vi "Write Sample Metadata.vi"(0 "File Path":path, 11 "Error In":errorcluster) -> (4 "File Path (Dup)":path, 8 "Canceled?":bool, 15 "Write Error":errorcluster)   [LabVIEW 2016]
uses:
  <vilib>/Utility/miscctls.llb/LVPointTypeDef.ctl
  Sampel Metadata Type Defs/Sample Metadata Full Data.ctl
  Sampel Metadata Type Defs/Sample Metadata Name Value Pair.ctl
  Sampel Metadata Type Defs/Sample Metadata Probe Data.ctl
  <vilib>/regexp/Match Regular Expression.xnode
  shell32.dll
panel:
  out "Current Path":string
  out "Last File Write Error":errorcluster
  in  "Dirty Quit":bool
  in  "Scavenger 06":u16(ring) items=["Not Applicable", "-", "Add Item"]
  in  "Scavenger 05":u16(ring) items=["Not Applicable", "-", "Add Item"]
  in  "Scavenger 04":u16(ring) items=["Not Applicable", "-", "Add Item"]
  in  "Scavenger 03":u16(ring) items=["Not Applicable", "-", "Add Item"]
  in  "Scavenger 02":u16(ring) items=["Not Applicable", "-", "Add Item"]
  in  "Scavenger 01":u16(ring) items=["Not Applicable", "-", "Add Item"]
  in  "Load Preset":bool
  in  "Sealant":u16(ring) items=["Not Applicable", "-", "Add Item"]
  in  "Sample Holder":u16(ring) items=["Not Applicable", "-", "Add Item"]
  in  "Preset Metadata":u16(ring) items=["None"]
  in  "Save New Preset":bool
  in  "Notes":string caption="Additional Notes (e.g. fixation info)"
  in  "Extra Tag 06":u16(ring) caption="Extra Tag" items=["Not Applicable", "-", "Add Item"]
  in  "Extra Tag 05":u16(ring) caption="Extra Tag" items=["Not Applicable", "-", "Add Item"]
  in  "Extra Tag 04":u16(ring) caption="Extra Tag" items=["Not Applicable", "-", "Add Item"]
  in  "Extra Tag 03":u16(ring) caption="Extra Tag" items=["Not Applicable", "-", "Add Item"]
  in  "Extra Tag 02":u16(ring) caption="Extra Tag" items=["Not Applicable", "-", "Add Item"]
  in  "Extra Tag 01":u16(ring) caption="Extra Tag" items=["Not Applicable", "-", "Add Item"]
  in  "Image Target 04":u16(ring) caption="Image Target" items=["Not Applicable", "-", "Add Item"]
  in  "Image Target 03":u16(ring) caption="Image Target" items=["Not Applicable", "-", "Add Item"]
  in  "Image Target 02":u16(ring) caption="Image Target" items=["Not Applicable", "-", "Add Item"]
  in  "Image Target 01":u16(ring) caption="Probe Target" items=["Not Applicable", "-", "Add Item"]
  in  "Buffer PH":dbl=1.0 caption="PH"
  in  "Buffer Type":u16(ring) items=["Not Applicable", "-", "Add Item"]
  in  "Probe Concentration 04":dbl=1.0 caption="Concentration"
  in  "Probe Concentration 03":dbl=1.0 caption="Concentration"
  in  "Probe Concentration 02":dbl=1.0 caption="Concentration"
  in  "Probe Concentration 01":dbl=1.0 caption="Concentration"
  in  "Probe Cat Num 04":u16(ring) caption="Probe Cat Num" items=["Not Applicable", "-", "Add Item"]
  in  "Probe Sub Type 04":u16(ring) caption="Probe Sub Type" items=["Not Applicable", "-", "Add Item"]
  in  "Probe Name 04":u16(ring) caption="Probe Name" items=["Not Applicable", "-", "Add Item"]
  in  "Probe 4":bool
  in  "Probe Cat Num 03":u16(ring) caption="Probe Cat Num" items=["Not Applicable", "-", "Add Item"]
  in  "Probe Cat Num 02":u16(ring) caption="Probe Cat Num" items=["Not Applicable", "-", "Add Item"]
  in  "Probe Cat Num 01":u16(ring) caption="Catalog Number" items=["Not Applicable", "-", "Add Item"]
  in  "Probe Sub Type 03":u16(ring) caption="Probe Sub Type" items=["Not Applicable", "-", "Add Item"]
  in  "Probe Sub Type 02":u16(ring) caption="Probe Sub Type" items=["Not Applicable", "-", "Add Item"]
  in  "Probe Sub Type 01":u16(ring) caption="Probe Sub Type" items=["Not Applicable", "-", "Add Item"]
  in  "Probe Name 03":u16(ring) caption="Probe Name" items=["Not Applicable", "-", "Add Item"]
  in  "Probe Name 02":u16(ring) caption="Probe Name" items=["Not Applicable", "-", "Add Item"]
  in  "Probe Name 01":u16(ring) caption="Probe Name" items=["Not Applicable", "-", "Add Item"]
  in  "Probe 3":bool
  in  "Probe 2":bool
  in  "Probe 1":bool
  in  "Sample Type Sub Types":u16(ring) caption="Sample Sub Type" items=["Not Applicable", "-", "Add Item"]
  in  "Sample Type":u16(ring) items=["Not Applicable", "-", "Add Item"]
  in  "Cancel":bool
  in  "Save":bool
  # "Sample Type"
  # "Sample Mounting"
  # "Buffer Information"
  # "Oxygen Scavenger Components"
  # "Probe Information"
  # "Probe Active"
  # "Additional Tags"
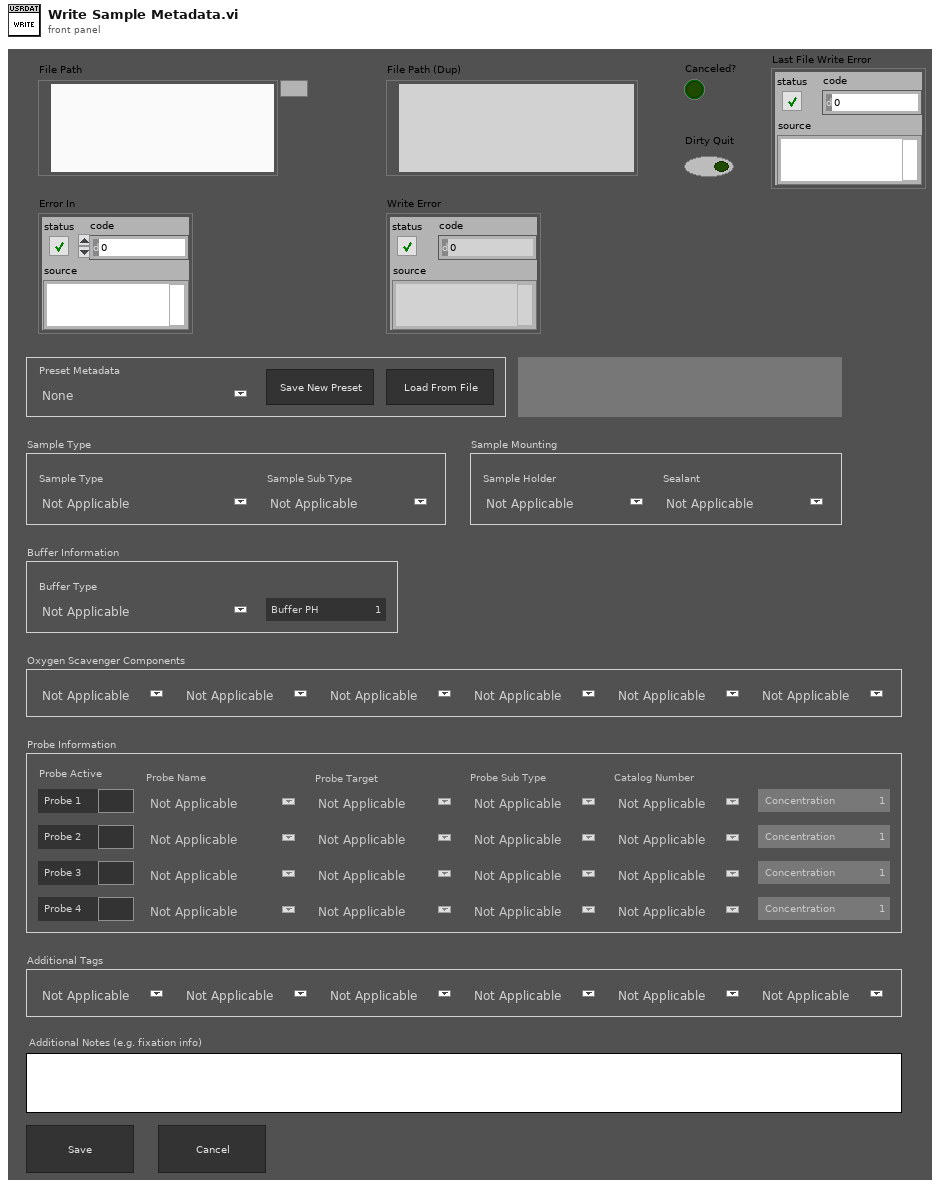
[diagram p1: front panel]
types:
  T1 = typedef "Sample Metadata Full Data.ctl" = cluster{"Sample Type":T2, "Sample Sub Type":T2, "Proble Data":T3[], "Buffer Type":T2, "Oxygen Scavenger":T2, "Buffer PH":dbl, "Extra Tags":T2[], "Sample Holder":T2, "Sealant":T2, "Notes":string, "Preset Name":string, "Scavenger Tags":T2[]}
  T2 = typedef "Sample Metadata Name Value Pair.ctl" = cluster{"String":string, "Value":u16}
  T3 = typedef "Sample Metadata Probe Data.ctl" = cluster{"Active?":bool, "Name":T2, "Target":T2, "Sub Type":T2, "Cat Number":T2, "Concentration":dbl}
  T4 = enum16{"Always On", "Always Off", "Off While Running"}
  T5 = typedef "LVPointTypeDef.ctl" = cluster{"Horizontal":i16, "Vertical":i16}
  T6 = enum8{"Enabled", "Disabled", "Disabled and Grayed Out"}
  T7 = typedef "LVRectTypeDef.ctl" = cluster{"Left":i16, "Top":i16, "Right":i16, "Bottom":i16}
  T8 = typedef "LVBoundsTypeDef.ctl" = cluster{"Width":u32, "Height":u32}
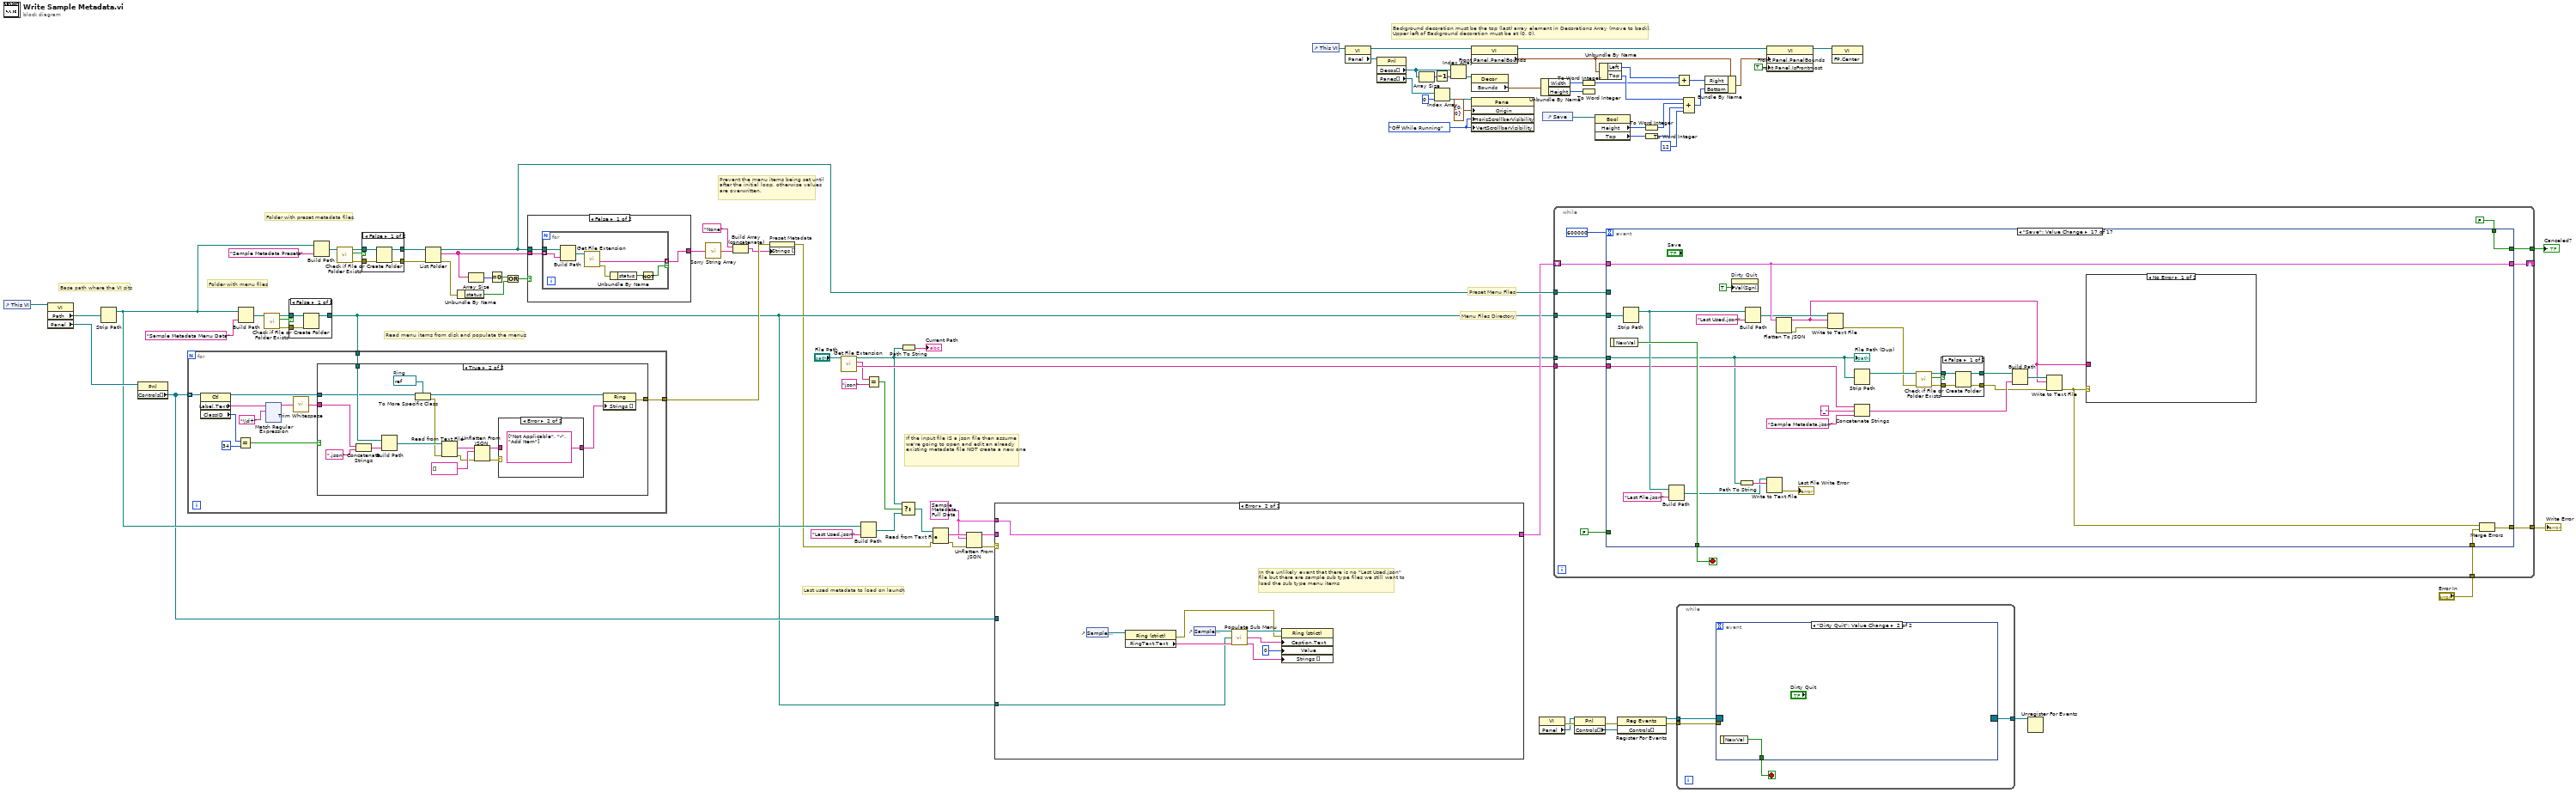
[diagram p0: block diagram]
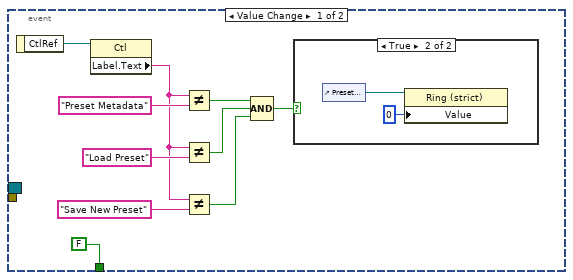
[diagram p2: hidden frame]
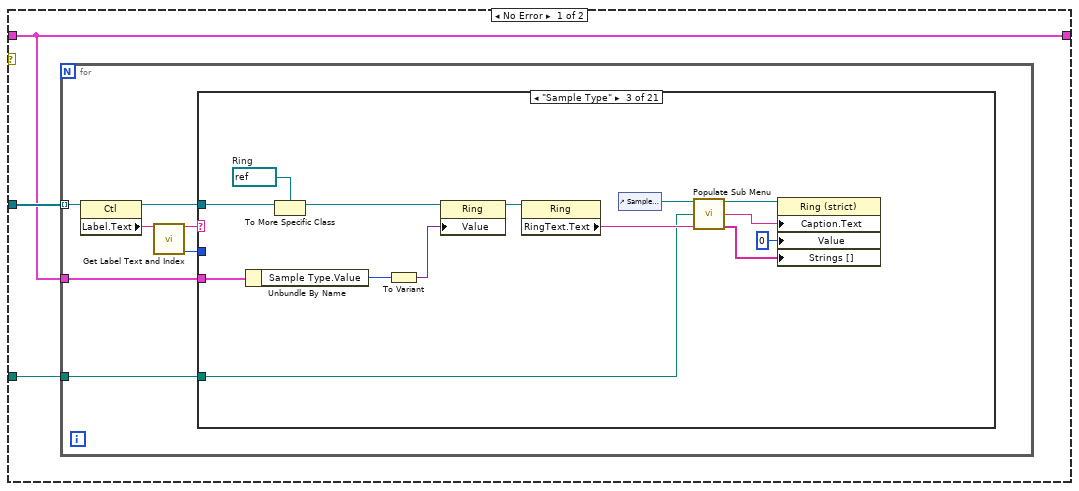
[diagram p4: hidden frame]
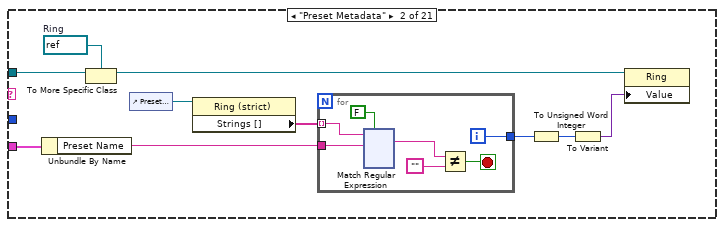
[diagram p6: hidden frame]
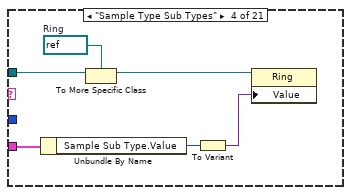
[diagram p7: hidden frame]
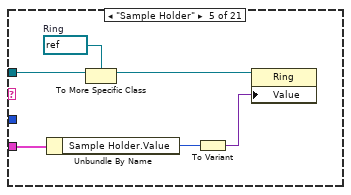
[diagram p8: hidden frame]
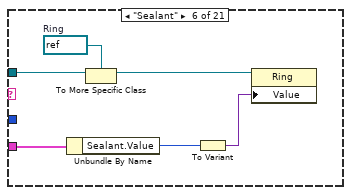
[diagram p9: hidden frame]
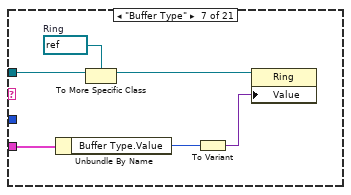
[diagram p10: hidden frame]
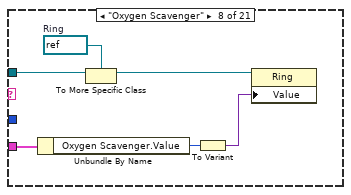
[diagram p11: hidden frame]
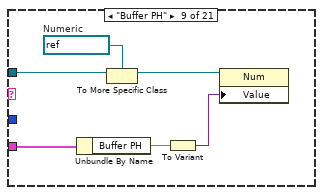
[diagram p12: hidden frame]
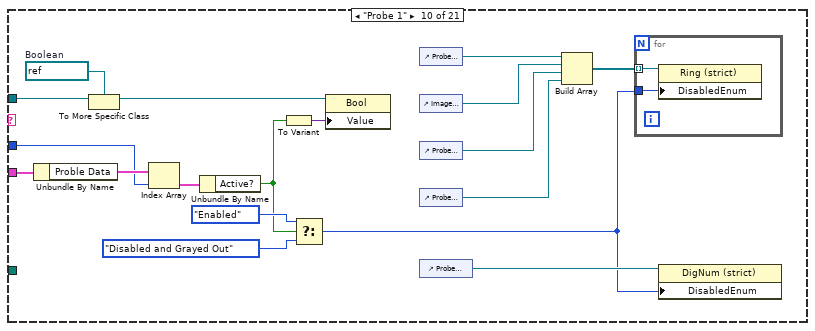
[diagram p13: hidden frame]
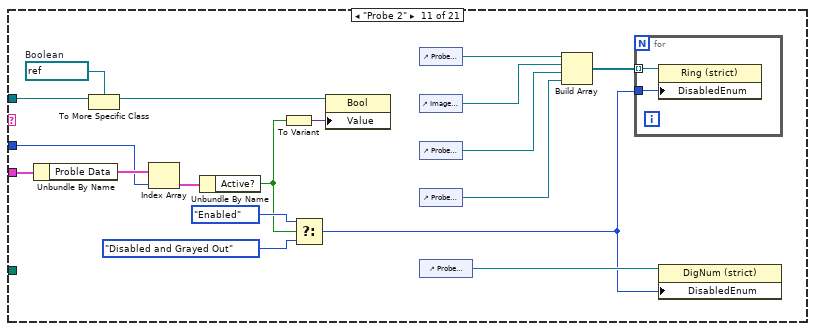
[diagram p14: hidden frame]
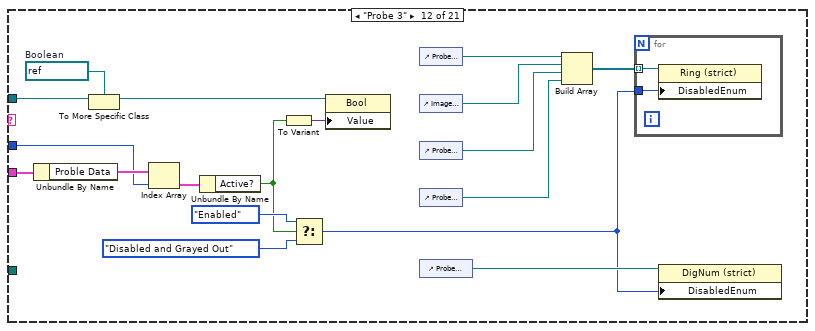
[diagram p15: hidden frame]
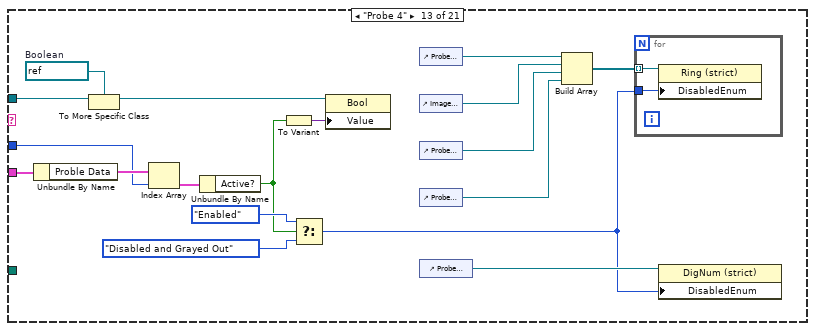
[diagram p16: hidden frame]
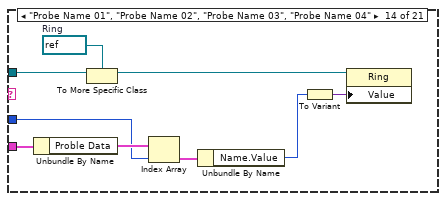
[diagram p17: hidden frame]
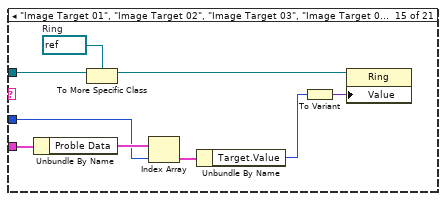
[diagram p18: hidden frame]
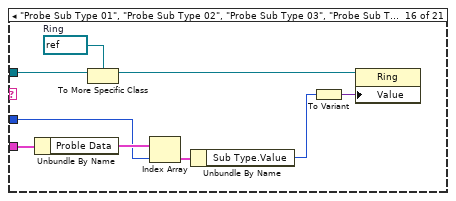
[diagram p19: hidden frame]
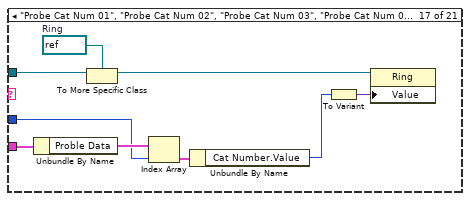
[diagram p20: hidden frame]
diagram:
  w29 = T1 {"Sample Type"={"String"="", "Value"=0}, "Sample Sub Type"={"String"="", "Value"=0}, "Proble Data"=[{"Active?"=FALSE, "Name"={"String"="", "Value"=0}, "Target"={"String"="", "Value"=0}, "Sub Type"={"String"="", "Value"=0}, "Cat Number"={"String"="", "Value"=0}, "Concentration"=0.0}, {"Active?"=FALSE, "Name"={"String"="", "Value"=0}, "Target"={"String"="", "Value"=0}, "Sub Type"={"String"="", "Value"=0}, "Cat Number"={"String"="", "Value"=0}, "Concentration"=0.0}, {"Active?"=FALSE, "Name"={"String"="", "Value"=0}, "Target"={"String"="", "Value"=0}, "Sub Type"={"String"="", "Value"=0}, "Cat Number"={"String"="", "Value"=0}, "Concentration"=0.0}, {"Active?"=FALSE, "Name"={"String"="", "Value"=0}, "Target"={"String"="", "Value"=0}, "Sub Type"={"String"="", "Value"=0}, "Cat Number"={"String"="", "Value"=0}, "Concentration"=0.0}], "Buffer Type"={"String"="", "Value"=0}, "Oxygen Scavenger"={"String"="", "Value"=0}, "Buffer PH"=0.0, "Extra Tags"=[{"String"="", "Value"=0}, {"String"="", "Value"=0}, {"String"="", "Value"=0}, {"String"="", "Value"=0}, {"String"="", "Value"=0}, {"String"="", "Value"=0}], "Sample Holder"={"String"="", "Value"=0}, "Sealant"={"String"="", "Value"=0}, "Notes"="", "Preset Name"="", "Scavenger Tags"=[{"String"="", "Value"=0}, {"String"="", "Value"=0}, {"String"="", "Value"=0}, {"String"="", "Value"=0}, {"String"="", "Value"=0}, {"String"="", "Value"=0}]} ("Sample Metadata")
  w71 = T4."Off While Running" ("Vertical Scrollbar Visibility")
  # "If the input file IS a json file then assume we're going to open and edit an already existing metadata file NOT create a new one"
  # "Last used metadata to load on launch"
  # "Preset Menu Files"
  # "Menu Files Directory"
  # "Prevent the menu items being set until after the initial loop, otherwise values are overwritten."
  # "Folder with preset metadata files"
  # "Folder with menu files"
  # "Read menu items from disk and populate the menus"
  # "Base path where the VI sits"
  # "Background decoration must be the top (last) array element in Decorations Array (move to back).\nUpper left of Background decoration must be at (0, 0)."
  n1 = control-ref of="This VI"() -> (w57:refnum<vi>)
  n2 = property class="VI"(reference=w57) -> ("Path"=w34:path, "Panel"=w55:refnum<vi>)  [unwired: 1 in, 2 out]
  n3 = Strip Path(path=w34) -> (stripped path=w33:path)  [unwired: 1 out]
  n4 = property class="Pnl"(reference=w55) -> ("Controls[]"=w28:refnum<vi>[])  [unwired: 1 in, 2 out]
  n5 = Build Path(base path=w33, name or relative path="Sample Metadata Menu Data") -> (appended path=w53:path)
  n6 = call <vilib>:"Check if File or Folder Exists.vi"("path"=w53) -> ("error out"=w38:errorcluster, "file or folder exists?"=w51:bool, "dup path"=w52:path)  [unwired: 8 in]
  n7 = case shown="False" w51 {
    tunnel: w52 -> [w91 w92]
    tunnel: [w90 w92] -> w26
    tunnel: w38 -> [w89 _]
    frame False {
      n8 = Create Folder(path (use dialog)=w91, error in=w89) -> (created path=w90:path)  [unwired: 1 in, 2 out]
    }
    frame True {
    }
  }
  n9 = for {
    tunnel: w28 -> [w103] mode=indexing
    tunnel: w26 -> [w99]
    tunnel: [w93] -> w37
    n10 = property class="Ctl"(reference=w103) -> (reference out=w101:refnum<vi>, "Label.Text"=w96:string, "ClassID"=w100:u32)  [unwired: 1 in, 1 out]
    n11 = Equal?(x=w100, y=u32 34) -> (x = y?=w102:bool)
    n12 = xnode "Match Regular Expression"("input string"=w96, "regular expression"="\\d+") -> ("before match"=w98:string)  [unwired: 4 in, 4 out]
    n13 = call <vilib>:"Trim Whitespace.vi"("string"=w98) -> ("trimmed string"=w95:string)  [unwired: 1 in]
    n14 = case shown="True" w102 {
      tunnel: w101 -> [_ w224]
      tunnel: w95 -> [_ w232]
      tunnel: w99 -> [_ w231]
      tunnel: [errorcluster {"status"=FALSE, "code"=0, "source"=""} ("error out") w219] -> w93
      frame False {
      }
      frame True {
        w223 = refnum<vi> refnum  # Ring
        n15 = Concatenate Strings(w232, ".json") -> (w233:string)
        n16 = Build Path(base path=w231, name or relative path=w233) -> (appended path=w230:path)
        n17 = To More Specific Class(target class=w223, reference=w224) -> (specific class reference=w222:refnum<vi>, error out=w220:errorcluster)  [unwired: 1 in]
        n18 = Read from Text File(file (use dialog)=w230, error in=w220) -> (text=w229:string, error out=w227:errorcluster)  [unwired: 2 in, 2 out]
        n19 = Unflatten From JSON(JSON string=w229, type and defaults=string[] [], error in (no error)=w227) -> (value=w225:string[], error out=w226:errorcluster)  [unwired: 4 in]
        n20 = case shown="Error" w226 {
          tunnel: w225 -> [w235 _]
          tunnel: [w235 string[] ["Not Applicable", "-", "Add Item"]] -> w221
          frame No Error {
          }
          frame Error {
          }
        }
        n21 = property class="Ring"(reference=w222, "Strings []"=w221) -> (error out=w219:errorcluster)  [unwired: 1 in, 1 out]
      }
    }
  }
  n22 = Build Path(base path=w33, name or relative path="Sample Metadata Presets") -> (appended path=w48:path)
  n23 = call <vilib>:"Check if File or Folder Exists.vi"("path"=w48) -> ("error out"=w40:errorcluster, "file or folder exists?"=w50:bool, "dup path"=w49:path)  [unwired: 8 in]
  n24 = case shown="False" w50 {
    tunnel: w49 -> [w240 w242]
    tunnel: [w239 w242] -> w47
    tunnel: w40 -> [w238 w241]
    tunnel: [w237 w241] -> w39
    frame False {
      n25 = Create Folder(path (use dialog)=w240, error in=w238) -> (created path=w239:path, error out=w237:errorcluster)  [unwired: 1 in, 1 out]
    }
    frame True {
    }
  }
  n26 = List Folder(path=w47, error in=w39) -> (path out=w36:path, filenames=w45:string[], error out=w46:errorcluster)  [unwired: 2 in, 1 out]
  n27 = Unbundle By Name(w46) -> ("status"=w42:bool)
  n28 = Array Size(array=w45) -> (size(s)=w44:i32)
  n29 = Equal To 0?(x=w44) -> (x = 0?=w43:bool)
  n30 = Or(x=w43, y=w42) -> (x .or. y?=w41:bool)
  n31 = case shown="False" w41 {
    tunnel: w45 -> [w245 _]
    tunnel: [w243 string[] []] -> w22
    tunnel: w36 -> [w244 _]
    frame False {
      n32 = for {
        tunnel: w245 -> [w251] mode=indexing
        tunnel: w244 -> [w252]
        tunnel: [w249] -> w243 mode=indexing if=w246
        n33 = Build Path(base path=w252, name or relative path=w251) -> (appended path=w250:path)
        n34 = call <vilib>:"Get File Extension.vi"("file"=w250) -> ("error out"=w248:errorcluster, "filename without extension"=w249:string)  [unwired: 6 in, 3 out]
        n35 = Unbundle By Name(w248) -> ("status"=w247:bool)
        n36 = Not(x=w247) -> (.not. x?=w246:bool)
      }
    }
    frame True {
    }
  }
  n37 = call "Sorry String Array.vi"("Array of String"=w22) -> ("Sorted Array"=w21:string[])  [unwired: 14 in]
  n38 = Build Array (concatenate)("None", w21) -> (w19:string[])
  n39 = property on="Preset Metadata" class="Ring (strict)"(error in=w37, "Strings []"=w19) -> (error out=w18:errorcluster)  [unwired: 1 in, 1 out]
  n40 = call <vilib>:"Get File Extension.vi"("file"="File Path") -> ("filename without extension"=w8:string, "lowercase file extension"=w7:string, "dup file"=w2:path)  [unwired: 6 in, 2 out]
  n41 = Build Path(base path=w33, name or relative path="Last Used.json") -> (appended path=w4:path)
  n42 = Equal?(x=w7, y="json") -> (x = y?=w5:bool)
  n43 = Select(t=w2, s=w5, f=w4) -> (s? t:f=w3:path)
  n44 = Path To String(path=w2) -> (string=→"Current Path":string)
  n45 = Read from Text File(file (use dialog)=w3, error in=w18) -> (text=w32:string, error out=w17:errorcluster)  [unwired: 2 in, 2 out]
  n46 = Unflatten From JSON(JSON string=w32, type and defaults=w29, error in (no error)=w17) -> (value=w30:T1, error out=w31:errorcluster)  [unwired: 4 in]
  n47 = case shown="Error" w31 {
    tunnel: [w254 w602] -> w27
    tunnel: w28 -> [w256 _]
    tunnel: w26 -> [w255 w594]
    tunnel: w30 -> [w254 _]
    tunnel: w29 -> [_ w602]
    frame No Error {
      n48 = for {
        tunnel: w256 -> [w263] mode=indexing
        tunnel: w254 -> [w261]
        tunnel: w255 -> [w260]
        n49 = property class="Ctl"(reference=w263) -> (reference out=w262:refnum<vi>, "Label.Text"=w259:string)  [unwired: 1 in, 1 out]
        n50 = call "Get Label Text and Index.vi"("Label Text and Index"=w259) -> ("Label Text and Index (Dup)"=w258:string, "Index"=w257:i32)  [unwired: 12 in, 1 out]
        n51 = case shown="\"Sample Type\"" w258 {
          tunnel: w262 -> [_ w272 w407 w413 w419 w425 w431 w437 w443 w458 w478 w498 w518 w530 w539 w548 w557 w566 w575 w584 w590]
          tunnel: w261 -> [_ w270 w405 w411 w417 w423 w429 w435 w441 w462 w482 w502 w522 w533 w542 w551 w560 w569 w578 w587 w589]
          tunnel: w260 -> [_ _ w395 _ _ _ _ _ _ _ _ _ _ _ _ _ _ _ _ _ _]
          tunnel: w257 -> [_ _ _ _ _ _ _ _ _ w445 w465 w485 w505 w525 w534 w543 w552 w561 w570 w579 _]
          frame Default {
          }
          frame "Preset Metadata" {
            w273 = refnum<vi> refnum  # Ring
            n52 = Unbundle By Name(w270) -> ("Preset Name"=w265:string)
            n53 = To More Specific Class(target class=w273, reference=w272) -> (specific class reference=w271:refnum<vi>)  [unwired: 1 in, 1 out]
            n54 = control-ref of="Preset Metadata"() -> (w267:refnum<vi>)
            n55 = property class="Ring (strict)"(reference=w267) -> ("Strings []"=w268:string[])  [unwired: 1 in, 2 out]
            n56 = for {
              tunnel: w265 -> [w280]
              tunnel: w268 -> [w278] mode=indexing
              tunnel: [w274] -> w266
              i -> [w274]
              stop <- w277 stop-if-true
              n57 = xnode "Match Regular Expression"("input string"=w278, "regular expression"=w280, "ignore case? (F)"=FALSE) -> ("whole match"=w276:string)  [unwired: 3 in, 4 out]
              n58 = Not Equal?(x=w276, y="") -> (x != y?=w277:bool)
            }
            n59 = To Unsigned Word Integer(number=w266) -> (unsigned 16bit integer=w264:u16)
            n60 = To Variant(anything=w264) -> (Variant=w269:variant)
            n61 = property class="Ring"(reference=w271, "Value"=w269) -> ()  [unwired: 1 in, 2 out]
          }
          frame "Sample Type" {
            w408 = refnum<vi> refnum  # Ring
            n62 = Unbundle By Name(w405) -> ("Sample Type.Value"=w404:u16)
            n63 = To More Specific Class(target class=w408, reference=w407) -> (specific class reference=w406:refnum<vi>)  [unwired: 1 in, 1 out]
            n64 = To Variant(anything=w404) -> (Variant=w403:variant)
            n65 = property class="Ring"(reference=w406, "Value"=w403) -> (reference out=w402:refnum<vi>)  [unwired: 1 in, 1 out]
            n66 = property class="Ring"(reference=w402) -> ("RingText.Text"=w396:string)  [unwired: 1 in, 2 out]
            n67 = control-ref of="Sample Type Sub Types"() -> (w400:refnum<vi>)
            n68 = call "Populate Sub Menu.vi"("Sample Type Sub Types"=w400, "Base Path"=w395, "Ring Text"=w396) -> ("Sample Type Sub Types (Dup)"=w399:refnum<vi>, "Caption Text"=w398:string, "Menu Items"=w397:string[])  [unwired: 10 in]
            n69 = property class="Ring (strict)"(reference=w399, "Caption.Text"=w398, "Value"=u16 0, "Strings []"=w397) -> ()  [unwired: 1 in, 2 out]
          }
          frame "Sample Type Sub Types" {
            w414 = refnum<vi> refnum  # Ring
            n70 = Unbundle By Name(w411) -> ("Sample Sub Type.Value"=w410:u16)
            n71 = To More Specific Class(target class=w414, reference=w413) -> (specific class reference=w412:refnum<vi>)  [unwired: 1 in, 1 out]
            n72 = To Variant(anything=w410) -> (Variant=w409:variant)
            n73 = property class="Ring"(reference=w412, "Value"=w409) -> ()  [unwired: 1 in, 2 out]
          }
          frame "Sample Holder" {
            w420 = refnum<vi> refnum  # Ring
            n74 = Unbundle By Name(w417) -> ("Sample Holder.Value"=w416:u16)
            n75 = To More Specific Class(target class=w420, reference=w419) -> (specific class reference=w418:refnum<vi>)  [unwired: 1 in, 1 out]
            n76 = To Variant(anything=w416) -> (Variant=w415:variant)
            n77 = property class="Ring"(reference=w418, "Value"=w415) -> ()  [unwired: 1 in, 2 out]
          }
          frame "Sealant" {
            w426 = refnum<vi> refnum  # Ring
            n78 = Unbundle By Name(w423) -> ("Sealant.Value"=w422:u16)
            n79 = To More Specific Class(target class=w426, reference=w425) -> (specific class reference=w424:refnum<vi>)  [unwired: 1 in, 1 out]
            n80 = To Variant(anything=w422) -> (Variant=w421:variant)
            n81 = property class="Ring"(reference=w424, "Value"=w421) -> ()  [unwired: 1 in, 2 out]
          }
          frame "Buffer Type" {
            w432 = refnum<vi> refnum  # Ring
            n82 = Unbundle By Name(w429) -> ("Buffer Type.Value"=w428:u16)
            n83 = To More Specific Class(target class=w432, reference=w431) -> (specific class reference=w430:refnum<vi>)  [unwired: 1 in, 1 out]
            n84 = To Variant(anything=w428) -> (Variant=w427:variant)
            n85 = property class="Ring"(reference=w430, "Value"=w427) -> ()  [unwired: 1 in, 2 out]
          }
          frame "Oxygen Scavenger" {
            w438 = refnum<vi> refnum  # Ring
            n86 = Unbundle By Name(w435) -> ("Oxygen Scavenger.Value"=w434:u16)
            n87 = To More Specific Class(target class=w438, reference=w437) -> (specific class reference=w436:refnum<vi>)  [unwired: 1 in, 1 out]
            n88 = To Variant(anything=w434) -> (Variant=w433:variant)
            n89 = property class="Ring"(reference=w436, "Value"=w433) -> ()  [unwired: 1 in, 2 out]
          }
          frame "Buffer PH" {
            w444 = refnum<vi> refnum  # Numeric
            n90 = Unbundle By Name(w441) -> ("Buffer PH"=w440:dbl)
            n91 = To More Specific Class(target class=w444, reference=w443) -> (specific class reference=w442:refnum<vi>)  [unwired: 1 in, 1 out]
            n92 = To Variant(anything=w440) -> (Variant=w439:variant)
            n93 = property class="Num"(reference=w442, "Value"=w439) -> ()  [unwired: 1 in, 2 out]
          }
          frame "Probe 1" {
            w459 = refnum<vi> refnum  # Boolean
            n94 = Unbundle By Name(w462) -> ("Proble Data"=w461:T3[])
            n95 = To More Specific Class(target class=w459, reference=w458) -> (specific class reference=w457:refnum<vi>)  [unwired: 1 in, 1 out]
            n96 = Index Array(array=w461, index=w445) -> (element=w460:T3)
            n97 = Unbundle By Name(w460) -> ("Active?"=w447:bool)
            n98 = To Variant(anything=w447) -> (Variant=w456:variant)
            n99 = Select(t=T6."Enabled" ("Disabled"), s=w447, f=T6."Disabled and Grayed Out" ("Disabled")) -> (s? t:f=w446:T6)
            n100 = property class="Bool"(reference=w457, "Value"=w456) -> ()  [unwired: 1 in, 2 out]
            n101 = control-ref of="Probe Name 01"() -> (w452:refnum<vi>)
            n102 = control-ref of="Image Target 01"() -> (w453:refnum<vi>)
            n103 = control-ref of="Probe Sub Type 01"() -> (w454:refnum<vi>)
            n104 = control-ref of="Probe Cat Num 01"() -> (w455:refnum<vi>)
            n105 = control-ref of="Probe Concentration 01"() -> (w450:refnum<vi>)
            n106 = Build Array(w452, w453, w454, w455) -> (w451:refnum<vi>[])
            n107 = for {
              tunnel: w451 -> [w464] mode=indexing
              tunnel: w446 -> [w463]
              n108 = property class="Ring (strict)"(reference=w464, "DisabledEnum"=w463) -> ()  [unwired: 1 in, 2 out]
            }
            n109 = property class="DigNum (strict)"(reference=w450, "DisabledEnum"=w446) -> ()  [unwired: 1 in, 2 out]
          }
          frame "Probe 2" {
            w479 = refnum<vi> refnum  # Boolean
            n110 = Unbundle By Name(w482) -> ("Proble Data"=w481:T3[])
            n111 = To More Specific Class(target class=w479, reference=w478) -> (specific class reference=w477:refnum<vi>)  [unwired: 1 in, 1 out]
            n112 = Index Array(array=w481, index=w465) -> (element=w480:T3)
            n113 = Unbundle By Name(w480) -> ("Active?"=w467:bool)
            n114 = To Variant(anything=w467) -> (Variant=w476:variant)
            n115 = Select(t=T6."Enabled" ("Disabled"), s=w467, f=T6."Disabled and Grayed Out" ("Disabled")) -> (s? t:f=w466:T6)
            n116 = property class="Bool"(reference=w477, "Value"=w476) -> ()  [unwired: 1 in, 2 out]
            n117 = control-ref of="Probe Name 02"() -> (w472:refnum<vi>)
            n118 = control-ref of="Image Target 02"() -> (w473:refnum<vi>)
            n119 = control-ref of="Probe Sub Type 02"() -> (w474:refnum<vi>)
            n120 = control-ref of="Probe Cat Num 02"() -> (w475:refnum<vi>)
            n121 = control-ref of="Probe Concentration 02"() -> (w470:refnum<vi>)
            n122 = Build Array(w472, w473, w474, w475) -> (w471:refnum<vi>[])
            n123 = for {
              tunnel: w471 -> [w484] mode=indexing
              tunnel: w466 -> [w483]
              n124 = property class="Ring (strict)"(reference=w484, "DisabledEnum"=w483) -> ()  [unwired: 1 in, 2 out]
            }
            n125 = property class="DigNum (strict)"(reference=w470, "DisabledEnum"=w466) -> ()  [unwired: 1 in, 2 out]
          }
          frame "Probe 3" {
            w499 = refnum<vi> refnum  # Boolean
            n126 = Unbundle By Name(w502) -> ("Proble Data"=w501:T3[])
            n127 = To More Specific Class(target class=w499, reference=w498) -> (specific class reference=w497:refnum<vi>)  [unwired: 1 in, 1 out]
            n128 = Index Array(array=w501, index=w485) -> (element=w500:T3)
            n129 = Unbundle By Name(w500) -> ("Active?"=w487:bool)
            n130 = To Variant(anything=w487) -> (Variant=w496:variant)
            n131 = Select(t=T6."Enabled" ("Disabled"), s=w487, f=T6."Disabled and Grayed Out" ("Disabled")) -> (s? t:f=w486:T6)
            n132 = property class="Bool"(reference=w497, "Value"=w496) -> ()  [unwired: 1 in, 2 out]
            n133 = control-ref of="Probe Name 03"() -> (w492:refnum<vi>)
            n134 = control-ref of="Image Target 03"() -> (w493:refnum<vi>)
            n135 = control-ref of="Probe Sub Type 03"() -> (w494:refnum<vi>)
            n136 = control-ref of="Probe Cat Num 03"() -> (w495:refnum<vi>)
            n137 = control-ref of="Probe Concentration 03"() -> (w490:refnum<vi>)
            n138 = Build Array(w492, w493, w494, w495) -> (w491:refnum<vi>[])
            n139 = for {
              tunnel: w491 -> [w504] mode=indexing
              tunnel: w486 -> [w503]
              n140 = property class="Ring (strict)"(reference=w504, "DisabledEnum"=w503) -> ()  [unwired: 1 in, 2 out]
            }
            n141 = property class="DigNum (strict)"(reference=w490, "DisabledEnum"=w486) -> ()  [unwired: 1 in, 2 out]
          }
          frame "Probe 4" {
            w519 = refnum<vi> refnum  # Boolean
            n142 = Unbundle By Name(w522) -> ("Proble Data"=w521:T3[])
            n143 = To More Specific Class(target class=w519, reference=w518) -> (specific class reference=w517:refnum<vi>)  [unwired: 1 in, 1 out]
            n144 = Index Array(array=w521, index=w505) -> (element=w520:T3)
            n145 = Unbundle By Name(w520) -> ("Active?"=w507:bool)
            n146 = To Variant(anything=w507) -> (Variant=w516:variant)
            n147 = Select(t=T6."Enabled" ("Disabled"), s=w507, f=T6."Disabled and Grayed Out" ("Disabled")) -> (s? t:f=w506:T6)
            n148 = property class="Bool"(reference=w517, "Value"=w516) -> ()  [unwired: 1 in, 2 out]
            n149 = control-ref of="Probe Name 04"() -> (w512:refnum<vi>)
            n150 = control-ref of="Image Target 04"() -> (w513:refnum<vi>)
            n151 = control-ref of="Probe Sub Type 04"() -> (w514:refnum<vi>)
            n152 = control-ref of="Probe Cat Num 04"() -> (w515:refnum<vi>)
            n153 = control-ref of="Probe Concentration 04"() -> (w510:refnum<vi>)
            n154 = Build Array(w512, w513, w514, w515) -> (w511:refnum<vi>[])
            n155 = for {
              tunnel: w511 -> [w524] mode=indexing
              tunnel: w506 -> [w523]
              n156 = property class="Ring (strict)"(reference=w524, "DisabledEnum"=w523) -> ()  [unwired: 1 in, 2 out]
            }
            n157 = property class="DigNum (strict)"(reference=w510, "DisabledEnum"=w506) -> ()  [unwired: 1 in, 2 out]
          }
          frame "Probe Name 01", "Probe Name 02", "Probe Name 03", "Probe Name 04" {
            w526 = refnum<vi> refnum  # Ring
            n158 = Unbundle By Name(w533) -> ("Proble Data"=w532:T3[])
            n159 = To More Specific Class(target class=w526, reference=w530) -> (specific class reference=w529:refnum<vi>)  [unwired: 1 in, 1 out]
            n160 = Index Array(array=w532, index=w525) -> (element=w531:T3)
            n161 = Unbundle By Name(w531) -> ("Name.Value"=w527:u16)
            n162 = To Variant(anything=w527) -> (Variant=w528:variant)
            n163 = property class="Ring"(reference=w529, "Value"=w528) -> ()  [unwired: 1 in, 2 out]
          }
          frame "Image Target 01", "Image Target 02", "Image Target 03", "Image Target 04" {
            w535 = refnum<vi> refnum  # Ring
            n164 = Unbundle By Name(w542) -> ("Proble Data"=w541:T3[])
            n165 = To More Specific Class(target class=w535, reference=w539) -> (specific class reference=w538:refnum<vi>)  [unwired: 1 in, 1 out]
            n166 = Index Array(array=w541, index=w534) -> (element=w540:T3)
            n167 = Unbundle By Name(w540) -> ("Target.Value"=w536:u16)
            n168 = To Variant(anything=w536) -> (Variant=w537:variant)
            n169 = property class="Ring"(reference=w538, "Value"=w537) -> ()  [unwired: 1 in, 2 out]
          }
          frame "Probe Sub Type 01", "Probe Sub Type 02", "Probe Sub Type 03", "Probe Sub Type 04" {
            w544 = refnum<vi> refnum  # Ring
            n170 = Unbundle By Name(w551) -> ("Proble Data"=w550:T3[])
            n171 = To More Specific Class(target class=w544, reference=w548) -> (specific class reference=w547:refnum<vi>)  [unwired: 1 in, 1 out]
            n172 = Index Array(array=w550, index=w543) -> (element=w549:T3)
            n173 = Unbundle By Name(w549) -> ("Sub Type.Value"=w545:u16)
            n174 = To Variant(anything=w545) -> (Variant=w546:variant)
            n175 = property class="Ring"(reference=w547, "Value"=w546) -> ()  [unwired: 1 in, 2 out]
          }
          frame "Probe Cat Num 01", "Probe Cat Num 02", "Probe Cat Num 03", "Probe Cat Num 04" {
            w553 = refnum<vi> refnum  # Ring
            n176 = Unbundle By Name(w560) -> ("Proble Data"=w559:T3[])
            n177 = To More Specific Class(target class=w553, reference=w557) -> (specific class reference=w556:refnum<vi>)  [unwired: 1 in, 1 out]
            n178 = Index Array(array=w559, index=w552) -> (element=w558:T3)
            n179 = Unbundle By Name(w558) -> ("Cat Number.Value"=w554:u16)
            n180 = To Variant(anything=w554) -> (Variant=w555:variant)
            n181 = property class="Ring"(reference=w556, "Value"=w555) -> ()  [unwired: 1 in, 2 out]
          }
          frame "Probe Concentration 01", "Probe Concentration 02", "Probe Concentration 03", "Probe Concentration 04" {
            w562 = refnum<vi> refnum  # Numeric
            n182 = Unbundle By Name(w569) -> ("Proble Data"=w568:T3[])
            n183 = To More Specific Class(target class=w562, reference=w566) -> (specific class reference=w565:refnum<vi>)  [unwired: 1 in, 1 out]
            n184 = Index Array(array=w568, index=w561) -> (element=w567:T3)
            n185 = Unbundle By Name(w567) -> ("Concentration"=w563:dbl)
            n186 = To Variant(anything=w563) -> (Variant=w564:variant)
            n187 = property class="Num"(reference=w565, "Value"=w564) -> ()  [unwired: 1 in, 2 out]
          }
          frame "Extra Tag 01", "Extra Tag 02", "Extra Tag 03", "Extra Tag 04", "Extra Tag 05", "Extra Tag 06" {
            w571 = refnum<vi> refnum  # Ring
            n188 = Unbundle By Name(w578) -> ("Extra Tags"=w577:T2[])
            n189 = To More Specific Class(target class=w571, reference=w575) -> (specific class reference=w574:refnum<vi>)  [unwired: 1 in, 1 out]
            n190 = Index Array(array=w577, index=w570) -> (element=w576:T2)
            n191 = Unbundle By Name(w576) -> ("Value"=w572:u16)
            n192 = To Variant(anything=w572) -> (Variant=w573:variant)
            n193 = property class="Ring"(reference=w574, "Value"=w573) -> ()  [unwired: 1 in, 2 out]
          }
          frame "Scavenger 01", "Scavenger 02", "Scavenger 03", "Scavenger 04", "Scavenger 05", "Scavenger 06" {
            w580 = refnum<vi> refnum  # Ring
            n194 = Unbundle By Name(w587) -> ("Scavenger Tags"=w586:T2[])
            n195 = To More Specific Class(target class=w580, reference=w584) -> (specific class reference=w583:refnum<vi>)  [unwired: 1 in, 1 out]
            n196 = Index Array(array=w586, index=w579) -> (element=w585:T2)
            n197 = Unbundle By Name(w585) -> ("Value"=w581:u16)
            n198 = To Variant(anything=w581) -> (Variant=w582:variant)
            n199 = property class="Ring"(reference=w583, "Value"=w582) -> ()  [unwired: 1 in, 2 out]
          }
          frame "Notes" {
            w591 = refnum<vi> refnum  # String
            n200 = Unbundle By Name(w589) -> ("Notes"=w588:string)
            n201 = To More Specific Class(target class=w591, reference=w590) -> (specific class reference=w592:refnum<vi>)  [unwired: 1 in, 1 out]
            n202 = property class="Str"(reference=w592, "Value"=w588) -> ()  [unwired: 1 in, 2 out]
          }
        }
      }
    }
    frame Error {
      # "In the unlikely event that there is no \"Last Used.json\" file but there are sample sub type files we still want to load the sub type menu items"
      n203 = control-ref of="Sample Type"() -> (w595:refnum<vi>)
      n204 = property class="Ring (strict)"(reference=w595) -> (error out=w593:errorcluster, "RingText.Text"=w596:string)  [unwired: 1 in, 1 out]
      n205 = control-ref of="Sample Type Sub Types"() -> (w600:refnum<vi>)
      n206 = call "Populate Sub Menu.vi"("Sample Type Sub Types"=w600, "Base Path"=w594, "Ring Text"=w596) -> ("Sample Type Sub Types (Dup)"=w599:refnum<vi>, "Caption Text"=w598:string, "Menu Items"=w597:string[])  [unwired: 10 in]
      n207 = property class="Ring (strict)"(reference=w599, error in=w593, "Caption.Text"=w598, "Value"=u16 0, "Strings []"=w597) -> ()  [unwired: 2 out]
    }
  }
  n208 = control-ref of="This VI"() -> (w63:refnum<vi>)
  n209 = property class="VI"(reference=w63) -> (reference out=w72:refnum<vi>, "Panel"=w64:refnum<vi>)  [unwired: 1 in, 1 out]
  n210 = property class="Pnl"(reference=w64) -> ("Decos[]"=w62:refnum<vi>[], "Panes[]"=w68:refnum<vi>[])  [unwired: 1 in, 2 out]
  n211 = Array Size(array=w62) -> (size(s)=w60:i32)
  n212 = Decrement(x=w60) -> (x-1=w61:i32)
  n213 = Index Array(array=w68, index=0) -> (element=w67:refnum<vi>)
  n214 = Index Array(array=w62, index=w61) -> (element=w70:refnum<vi>)
  n215 = property class="VI"(reference=w72) -> (reference out=w74:refnum<vi>, "Front Panel.PanelBounds"=w75:T7)  [unwired: 1 in, 1 out]
  n216 = property class="Decor"(reference=w70) -> ("Bounds"=w73:T8)  [unwired: 1 in, 2 out]
  n217 = property class="Pane"(reference=w67, "Origin"=T5 {"Horizontal"=0, "Vertical"=0}, "HorizScrollbarVisibility"=w71, "VertScrollbarVisibility"=w71) -> ()  [unwired: 1 in, 2 out]
  n218 = property class="VI"() -> (error out=w16:errorcluster, "Panel"=w15:refnum<vi>)  [unwired: 2 in, 1 out]
  n219 = Unbundle By Name(w73) -> ("Width"=w78:u32, "Height"=w81:u32)
  n220 = control-ref of="Save"() -> (w65:refnum<vi>)
  n221 = while {
    tunnel: w26 -> [w614]
    shift-right: [w611] -> _
    shift-left: w27 -> [w612]
    tunnel: w36 -> [w610]
    tunnel: "Error In" -> [w608]
    tunnel: [w609] -> w24
    tunnel: [w605] -> w23
    tunnel: w2 -> [w604]
    tunnel: w8 -> [w603]
    stop <- w607 stop-if-true
    n222 = event shown="[16] \"Save\": Value Change" {
      selector: _ -> [_ _ _ _ _ _ _ _ _ _ _ _ _ _ _ _ _]
      dyn-events: _ -> [_ _ _ _ _ _ _ _ _ _ _ _ _ _ _ _ _]
      timeout: 600000 -> [_ _ _ _ _ _ _ _ _ _ _ _ _ _ _ _ _]
      tunnel: [TRUE ("NewVal") w635 w718 w754 w807 w854 w901 w948 w993 w1040 w1085 w1101 w1132 w1138 w1159 w1524 w1696] -> w607
      tunnel: w614 -> [_ w630 w713 _ w803 w850 w897 w944 w989 w1036 _ w1094 _ _ w1149 _ w1679]
      tunnel: FALSE -> [_ w635 w718 w754 w807 w854 w901 w948 w993 w1040 w1085 w1101 w1132 w1138 w1159 w1524 _]
      tunnel: w612 -> [w619 w627 w709 w745 w796 w843 w890 w937 w984 w1031 w1080 w1091 w1131 w1137 w1140 w1519 w1694]
      tunnel: [w619 w626 w708 w743 w795 w842 w889 w936 w983 w1030 w1079 w1090 w1129 w1135 w1148 w1518 w1694] -> w611
      tunnel: w610 -> [_ _ _ _ _ _ _ _ _ _ _ _ _ _ w1158 w1523 _]
      tunnel: [w618 w623 w704 w738 w786 w833 w880 w927 w974 w1021 w1068 w1087 w1128 w1134 w1147 w1517 w1688] -> w609
      tunnel: w608 -> [w618 w623 w704 w738 w786 w833 w880 w927 w974 w1021 w1068 w1087 w1128 w1134 w1147 w1517 w1689]
      tunnel: FALSE -> [_ w622 w703 w737 w785 w832 w879 w926 w973 w1020 w1067 w1086 w1127 w1133 w1146 w1516 w1687]
      tunnel: [TRUE w622 w703 w737 w785 w832 w879 w926 w973 w1020 w1067 w1086 w1127 w1133 w1146 w1516 w1687] -> w605
      tunnel: w604 -> [_ _ _ _ _ _ _ _ _ _ _ _ _ _ _ _ w1667]
      tunnel: w603 -> [_ _ _ _ _ _ _ _ _ _ _ _ _ _ _ _ w1668]
      event Timeout; "Cancel": Value Change {
        n223 = event-data() -> ()  [unwired: 1 in, 3 out]
        n224 = property on="Dirty Quit" class="Bool (strict)"("Val(Sgnl)"=TRUE ("Value (Signaling)")) -> ()  [unwired: 2 in, 2 out]
      }
      event "Sample Type": Value Change {
        n225 = event-data() -> ("OldVal"=w629:u16, "CtlRef"=w634:refnum<vi>)  [unwired: 1 in]
        n226 = property class="Ring (strict)"(reference=w634) -> (reference out=w631:refnum<vi>, "Label.Text"=w628:string, "RingText.Text"=w625:string, "Value"=w624:u16)  [unwired: 1 in, 1 out]
        n227 = control-ref of="Sample Type Sub Types"() -> (w621:refnum<vi>)
        n228 = Equal?(x=w625, y="Add Item") -> (x = y?=w632:bool)
        n229 = case shown="False" w632 {
          tunnel: w631 -> [_ w662]
          tunnel: w630 -> [w646 w655]
          tunnel: w629 -> [_ w663]
          tunnel: w628 -> [_ w661]
          tunnel: w625 -> [w640 _]
          tunnel: w627 -> [w642 w660]
          tunnel: [w641 w659] -> w626
          tunnel: w624 -> [w639 _]
          tunnel: w621 -> [w636 w649]
          frame False {
            n230 = call "Populate Sub Menu.vi"("Sample Type Sub Types"=w636, "Base Path"=w646, "Ring Text"=w640) -> ("Sample Type Sub Types (Dup)"=w645:refnum<vi>, "Caption Text"=w644:string, "Menu Items"=w643:string[])  [unwired: 10 in]
            n231 = Bundle(cluster=T2 {"String"="", "Value"=0} ("Name Value Pair"), "String"=w640, "Value"=w639) -> (w638:T2)
            n232 = property class="Ring (strict)"(reference=w645, "Caption.Text"=w644, "Value"=u16 0, "Strings []"=w643) -> ()  [unwired: 1 in, 2 out]
            n233 = Bundle By Name(cluster=w642, "Sample Type"=w638) -> (w641:T1)
          }
          frame True {
            n234 = call "Add New Menu Item.vi"("Base Path"=w655, "Old Value"=w663, "Ring Menu Ref"=w662, "Label or Caption"=w661) -> ("New Item"=w648:string, "Menu Value"=w658:u16)  [unwired: 8 in, 2 out]
            n235 = Concatenate Strings("Enter " ("string"), w648, " Sub Type Name") -> (w654:string)
            n236 = call "Get User Input.vi"("Dialog Message"=w654) -> ("User Input"=w651:string, "Canceled?"=w652:bool)  [unwired: 13 in]
            n237 = case shown="False" w652 {
              tunnel: w655 -> [w688 _]
              tunnel: w651 -> [w682 _]
              tunnel: w649 -> [w689 _]
              tunnel: w648 -> [w676 _]
              frame False {
                w671 = string[][] []
                w683 = string[] ["Not Applicable", "-", "Add Item"]
                n238 = Build Array(w676, w682) -> (w681:string[])
                n239 = property class="Ring (strict)"(reference=w689, "Value"=u16 0, "Caption.Text"=w682, "Strings []"=w683) -> ("Label.Text"=w685:string)  [unwired: 1 in, 2 out]
                n240 = Concatenate Strings(w685, ".json" ("string")) -> (w686:string)
                n241 = Build Path(base path=w688, name or relative path=w685) -> (appended path=w666:path)
                n242 = Build Path(base path=w688, name or relative path=w686) -> (appended path=w677:path)
                n243 = call <vilib>:"Check if File or Folder Exists.vi"("path"=w666) -> ("error out"=w669:errorcluster, "file or folder exists?"=w667:bool, "dup path"=w668:path)  [unwired: 8 in]
                n244 = Read from Text File(file (use dialog)=w677) -> (text=w684:string, error out=w679:errorcluster)  [unwired: 3 in, 2 out]
                n245 = case shown="False" w667 {
                  tunnel: w668 -> [w698 w700]
                  tunnel: [w697 w700] -> w665
                  tunnel: w669 -> [w696 w699]
                  tunnel: [w695 w699] -> w664
                  frame False {
                    n246 = Create Folder(path (use dialog)=w698, error in=w696) -> (created path=w697:path, error out=w695:errorcluster)  [unwired: 1 in, 1 out]
                  }
                  frame True {
                  }
                }
                n247 = Unflatten From JSON(JSON string=w684, type and defaults=w671, error in (no error)=w679) -> (value=w673:string[][], error out=w674:errorcluster)  [unwired: 4 in]
                n248 = Concatenate Strings(w682, ".json" ("string")) -> (w693:string)
                n249 = case shown="No Error" w674 {
                  tunnel: [w701 w702] -> w672
                  tunnel: w673 -> [w701 _]
                  tunnel: w671 -> [_ w702]
                  frame No Error {
                  }
                  frame Error {
                  }
                }
                n250 = Build Path(base path=w665, name or relative path=w693) -> (appended path=w692:path)
                n251 = Flatten To JSON(anything=w683, error in (no error)=w664) -> (JSON string=w691:string, 11:w690:errorcluster)  [unwired: 1 in]
                n252 = Build Array (concatenate)(w672, w681) -> (w680:string[][])
                n253 = Flatten To JSON(anything=w680) -> (JSON string=w678:string, 11:w675:errorcluster)  [unwired: 2 in]
                n254 = Write to Text File(file (use dialog)=w692, text=w691, error in=w690) -> ()  [unwired: 1 in, 3 out]
                n255 = Write to Text File(file (use dialog)=w677, text=w678, error in=w675) -> ()  [unwired: 1 in, 3 out]
              }
              frame True {
              }
            }
            n256 = Bundle(cluster=T2 {"String"="", "Value"=0} ("Name Value Pair"), "String"=w648, "Value"=w658) -> (w657:T2)
            n257 = Bundle By Name(cluster=w660, "Sample Type"=w657) -> (w659:T1)
          }
        }
      }
      event "Sample Type Sub Types": Value Change {
        n258 = event-data() -> ("OldVal"=w712:u16, "CtlRef"=w716:refnum<vi>)  [unwired: 1 in]
        n259 = property class="Ring (strict)"(reference=w716) -> (reference out=w714:refnum<vi>, "Label.Text"=w710:string, "Caption.Text"=w711:string, "RingText.Text"=w707:string, "Value"=w706:u16)  [unwired: 1 in, 1 out]
        n260 = Equal?(x=w707, y="Add Item") -> (x = y?=w715:bool)
        n261 = case shown="True" w715 {
          tunnel: w714 -> [_ w736]
          tunnel: w713 -> [_ w734]
          tunnel: w712 -> [_ w735]
          tunnel: w711 -> [_ w733]
          tunnel: w710 -> [_ w732]
          tunnel: w709 -> [w724 w730]
          tunnel: [w723 w729] -> w708
          tunnel: w707 -> [w722 _]
          tunnel: w706 -> [w721 _]
          tunnel: T2 {"String"="", "Value"=0} ("Name Value Pair") -> [w719 w725]
          frame False {
            n262 = Bundle(cluster=w719, "String"=w722, "Value"=w721) -> (w720:T2)
            n263 = Bundle By Name(cluster=w724, "Sample Sub Type"=w720) -> (w723:T1)
          }
          frame True {
            n264 = Build Path(base path=w734, name or relative path=w732) -> (appended path=w731:path)
            n265 = call "Add New Menu Item.vi"("Base Path"=w731, "Old Value"=w735, "Ring Menu Ref"=w736, "Label or Caption"=w733) -> ("New Item"=w728:string, "Menu Value"=w727:u16)  [unwired: 8 in, 2 out]
            n266 = Bundle(cluster=w725, "String"=w728, "Value"=w727) -> (w726:T2)
            n267 = Bundle By Name(cluster=w730, "Sample Sub Type"=w726) -> (w729:T1)
          }
        }
      }
      event "Probe 1", "Probe 2", "Probe 3", "Probe 4": Value Change {
        n268 = event-data() -> ("CtlRef"=w753:refnum<vi>, "NewVal"=w742:bool)  [unwired: 1 in]
        n269 = property class="Bool (strict)"(reference=w753) -> ("Label.Text"=w752:string)  [unwired: 1 in, 2 out]
        n270 = Select(t=T6."Enabled" ("Disabled"), s=w742, f=T6."Disabled and Grayed Out" ("Disabled")) -> (s? t:f=w739:T6)
        n271 = case shown="\"Probe 2\"" w752 {
          tunnel: [w760 w767 w774 w781] -> w749
          tunnel: [0 1 2 3] -> w741
          tunnel: [w758 w765 w772 w779] -> w740
          frame "Probe 1", Default {
            n272 = control-ref of="Probe Name 01"() -> (w763:refnum<vi>)
            n273 = control-ref of="Probe Sub Type 01"() -> (w762:refnum<vi>)
            n274 = control-ref of="Probe Cat Num 01"() -> (w761:refnum<vi>)
            n275 = control-ref of="Probe Concentration 01"() -> (w758:refnum<vi>)
            n276 = control-ref of="Image Target 01"() -> (w757:refnum<vi>)
            n277 = Build Array(w763, w762, w761, w757) -> (w760:refnum<vi>[])
          }
          frame "Probe 2" {
            n278 = control-ref of="Probe Name 02"() -> (w770:refnum<vi>)
            n279 = control-ref of="Probe Sub Type 02"() -> (w769:refnum<vi>)
            n280 = control-ref of="Probe Cat Num 02"() -> (w768:refnum<vi>)
            n281 = control-ref of="Probe Concentration 02"() -> (w765:refnum<vi>)
            n282 = control-ref of="Image Target 02"() -> (w764:refnum<vi>)
            n283 = Build Array(w770, w769, w768, w764) -> (w767:refnum<vi>[])
          }
          frame "Probe 3" {
            n284 = control-ref of="Probe Name 03"() -> (w777:refnum<vi>)
            n285 = control-ref of="Probe Sub Type 03"() -> (w776:refnum<vi>)
            n286 = control-ref of="Probe Cat Num 03"() -> (w775:refnum<vi>)
            n287 = control-ref of="Probe Concentration 03"() -> (w772:refnum<vi>)
            n288 = control-ref of="Image Target 03"() -> (w771:refnum<vi>)
            n289 = Build Array(w777, w776, w775, w771) -> (w774:refnum<vi>[])
          }
          frame "Probe 4" {
            n290 = control-ref of="Probe Name 04"() -> (w784:refnum<vi>)
            n291 = control-ref of="Probe Sub Type 04"() -> (w783:refnum<vi>)
            n292 = control-ref of="Probe Cat Num 04"() -> (w782:refnum<vi>)
            n293 = control-ref of="Probe Concentration 04"() -> (w779:refnum<vi>)
            n294 = control-ref of="Image Target 04"() -> (w778:refnum<vi>)
            n295 = Build Array(w784, w783, w782, w778) -> (w781:refnum<vi>[])
          }
        }
        n296 = property class="DigNum (strict)"(reference=w740, "DisabledEnum"=w739) -> ()  [unwired: 1 in, 2 out]
        n297 = for {
          tunnel: w749 -> [w756] mode=indexing
          tunnel: w739 -> [w755]
          n298 = property class="Ring (strict)"(reference=w756, "DisabledEnum"=w755) -> ()  [unwired: 1 in, 2 out]
        }
        n299 = Unbundle By Name(w745) -> ("Proble Data"=w747:T3[])
        n300 = Index Array(array=w747, index=w741) -> (element=w748:T3)
        n301 = Bundle By Name(cluster=w748, "Active?"=w742) -> (w746:T3)
        n302 = Replace Array Subset(array=w747, new element=w746, index=w741) -> (w744:T3[])
        n303 = Bundle By Name(cluster=w745, "Proble Data"=w744) -> (w743:T1)
      }
      event "Probe Name 01", "Probe Name 02", "Probe Name 03", "Probe Name 04": Value Change {
        n304 = event-data() -> ("OldVal"=w802:u16, "CtlRef"=w801:refnum<vi>)  [unwired: 1 in]
        n305 = property class="Ring (strict)"(reference=w801) -> (reference out=w804:refnum<vi>, "Label.Text"=w789:string, "RingText.Text"=w792:string, "Value"=w791:u16)  [unwired: 1 in, 1 out]
        n306 = call "Get Label Text and Index.vi"("Label Text and Index"=w789) -> ("Text"=w787:string, "Index"=w788:i32)  [unwired: 12 in, 1 out]
        n307 = Equal?(x=w792, y="Add Item") -> (x = y?=w805:bool)
        n308 = case shown="True" w805 {
          tunnel: w804 -> [_ w829]
          tunnel: w803 -> [_ w827]
          tunnel: w802 -> [_ w828]
          tunnel: [w808 w814] -> w794
          tunnel: [w809 w816] -> w793
          tunnel: w792 -> [w811 _]
          tunnel: w791 -> [w810 _]
          tunnel: T2 {"String"="", "Value"=0} ("Name Value Pair") -> [w812 w815]
          tunnel: w787 -> [_ w813]
          tunnel: w788 -> [w808 w814]
          frame False {
            n309 = Bundle(cluster=w812, "String"=w811, "Value"=w810) -> (w809:T2)
          }
          frame True {
            n310 = control-ref of="Probe Name 01"() -> (w822:refnum<vi>)
            n311 = control-ref of="Probe Name 02"() -> (w825:refnum<vi>)
            n312 = control-ref of="Probe Name 03"() -> (w824:refnum<vi>)
            n313 = control-ref of="Probe Name 04"() -> (w823:refnum<vi>)
            n314 = call "Add New Menu Item.vi"("Base Path"=w827, "Old Value"=w828, "Ring Menu Ref"=w829, "Label or Caption"=w813) -> ("Menu Strings"=w826:string[], "New Item"=w817:string, "Menu Value"=w818:u16)  [unwired: 8 in, 1 out]
            n315 = Bundle(cluster=w815, "String"=w817, "Value"=w818) -> (w816:T2)
            n316 = Build Array(w822, w825, w824, w823) -> (w821:refnum<vi>[])
            n317 = Delete From Array(array=w821, length=1, index=w814) -> (array with subset deleted=w819:refnum<vi>[])  [unwired: 1 out]
            n318 = for {
              tunnel: w819 -> [w831] mode=indexing
              tunnel: w826 -> [w830]
              n319 = property class="Ring (strict)"(reference=w831, "Strings []"=w830) -> ()  [unwired: 1 in, 2 out]
            }
          }
        }
        n320 = Unbundle By Name(w796) -> ("Proble Data"=w799:T3[])
        n321 = Index Array(array=w799, index=w794) -> (element=w800:T3)
        n322 = Bundle By Name(cluster=w800, "Name"=w793) -> (w798:T3)
        n323 = Replace Array Subset(array=w799, new element=w798, index=w794) -> (w797:T3[])
        n324 = Bundle By Name(cluster=w796, "Proble Data"=w797) -> (w795:T1)
      }
      event "Image Target 01", "Image Target 02", "Image Target 03", "Image Target 04": Value Change {
        n325 = event-data() -> ("OldVal"=w849:u16, "CtlRef"=w848:refnum<vi>)  [unwired: 1 in]
        n326 = property class="Ring (strict)"(reference=w848) -> (reference out=w851:refnum<vi>, "Label.Text"=w836:string, "RingText.Text"=w839:string, "Value"=w838:u16)  [unwired: 1 in, 1 out]
        n327 = call "Get Label Text and Index.vi"("Label Text and Index"=w836) -> ("Text"=w834:string, "Index"=w835:i32)  [unwired: 12 in, 1 out]
        n328 = Equal?(x=w839, y="Add Item") -> (x = y?=w852:bool)
        n329 = case shown="True" w852 {
          tunnel: w851 -> [_ w876]
          tunnel: w850 -> [_ w874]
          tunnel: w849 -> [_ w875]
          tunnel: [w855 w860] -> w841
          tunnel: [w856 w863] -> w840
          tunnel: w839 -> [w858 _]
          tunnel: w838 -> [w857 _]
          tunnel: T2 {"String"="", "Value"=0} ("Name Value Pair") -> [w859 w862]
          tunnel: w834 -> [_ w861]
          tunnel: w835 -> [w855 w860]
          frame False {
            n330 = Bundle(cluster=w859, "String"=w858, "Value"=w857) -> (w856:T2)
          }
          frame True {
            n331 = control-ref of="Image Target 01"() -> (w869:refnum<vi>)
            n332 = control-ref of="Image Target 02"() -> (w872:refnum<vi>)
            n333 = control-ref of="Image Target 03"() -> (w871:refnum<vi>)
            n334 = control-ref of="Image Target 04"() -> (w870:refnum<vi>)
            n335 = call "Add New Menu Item.vi"("Base Path"=w874, "Old Value"=w875, "Ring Menu Ref"=w876, "Label or Caption"=w861) -> ("Menu Strings"=w873:string[], "New Item"=w864:string, "Menu Value"=w865:u16)  [unwired: 8 in, 1 out]
            n336 = Bundle(cluster=w862, "String"=w864, "Value"=w865) -> (w863:T2)
            n337 = Build Array(w869, w872, w871, w870) -> (w868:refnum<vi>[])
            n338 = Delete From Array(array=w868, length=1, index=w860) -> (array with subset deleted=w866:refnum<vi>[])  [unwired: 1 out]
            n339 = for {
              tunnel: w866 -> [w878] mode=indexing
              tunnel: w873 -> [w877]
              n340 = property class="Ring (strict)"(reference=w878, "Strings []"=w877) -> ()  [unwired: 1 in, 2 out]
            }
          }
        }
        n341 = Unbundle By Name(w843) -> ("Proble Data"=w846:T3[])
        n342 = Index Array(array=w846, index=w841) -> (element=w847:T3)
        n343 = Bundle By Name(cluster=w847, "Target"=w840) -> (w845:T3)
        n344 = Replace Array Subset(array=w846, new element=w845, index=w841) -> (w844:T3[])
        n345 = Bundle By Name(cluster=w843, "Proble Data"=w844) -> (w842:T1)
      }
      event "Probe Sub Type 01", "Probe Sub Type 02", "Probe Sub Type 03", "Probe Sub Type 04": Value Change {
        n346 = event-data() -> ("OldVal"=w896:u16, "CtlRef"=w895:refnum<vi>)  [unwired: 1 in]
        n347 = property class="Ring (strict)"(reference=w895) -> (reference out=w898:refnum<vi>, "Label.Text"=w883:string, "RingText.Text"=w886:string, "Value"=w885:u16)  [unwired: 1 in, 1 out]
        n348 = call "Get Label Text and Index.vi"("Label Text and Index"=w883) -> ("Text"=w881:string, "Index"=w882:i32)  [unwired: 12 in, 1 out]
        n349 = Equal?(x=w886, y="Add Item") -> (x = y?=w899:bool)
        n350 = case shown="True" w899 {
          tunnel: w898 -> [_ w923]
          tunnel: w897 -> [_ w920]
          tunnel: w896 -> [_ w922]
          tunnel: w881 -> [_ w921]
          tunnel: [w902 w907] -> w888
          tunnel: [w903 w909] -> w887
          tunnel: w886 -> [w905 _]
          tunnel: w885 -> [w904 _]
          tunnel: T2 {"String"="", "Value"=0} ("Name Value Pair") -> [w906 w908]
          tunnel: w882 -> [w902 w907]
          frame False {
            n351 = Bundle(cluster=w906, "String"=w905, "Value"=w904) -> (w903:T2)
          }
          frame True {
            n352 = control-ref of="Probe Sub Type 01"() -> (w915:refnum<vi>)
            n353 = control-ref of="Probe Sub Type 02"() -> (w918:refnum<vi>)
            n354 = control-ref of="Probe Sub Type 03"() -> (w917:refnum<vi>)
            n355 = control-ref of="Probe Sub Type 04"() -> (w916:refnum<vi>)
            n356 = call "Add New Menu Item.vi"("Base Path"=w920, "Old Value"=w922, "Ring Menu Ref"=w923, "Label or Caption"=w921) -> ("Menu Strings"=w919:string[], "New Item"=w910:string, "Menu Value"=w911:u16)  [unwired: 8 in, 1 out]
            n357 = Bundle(cluster=w908, "String"=w910, "Value"=w911) -> (w909:T2)
            n358 = Build Array(w915, w918, w917, w916) -> (w914:refnum<vi>[])
            n359 = Delete From Array(array=w914, length=1, index=w907) -> (array with subset deleted=w912:refnum<vi>[])  [unwired: 1 out]
            n360 = for {
              tunnel: w912 -> [w925] mode=indexing
              tunnel: w919 -> [w924]
              n361 = property class="Ring (strict)"(reference=w925, "Strings []"=w924) -> ()  [unwired: 1 in, 2 out]
            }
          }
        }
        n362 = Unbundle By Name(w890) -> ("Proble Data"=w893:T3[])
        n363 = Index Array(array=w893, index=w888) -> (element=w894:T3)
        n364 = Bundle By Name(cluster=w894, "Sub Type"=w887) -> (w892:T3)
        n365 = Replace Array Subset(array=w893, new element=w892, index=w888) -> (w891:T3[])
        n366 = Bundle By Name(cluster=w890, "Proble Data"=w891) -> (w889:T1)
      }
      event "Probe Cat Num 01", "Probe Cat Num 02", "Probe Cat Num 03", "Probe Cat Num 04": Value Change {
        n367 = event-data() -> ("OldVal"=w943:u16, "CtlRef"=w942:refnum<vi>)  [unwired: 1 in]
        n368 = property class="Ring (strict)"(reference=w942) -> (reference out=w945:refnum<vi>, "Label.Text"=w931:string, "RingText.Text"=w930:string, "Value"=w933:u16)  [unwired: 1 in, 1 out]
        n369 = call "Get Label Text and Index.vi"("Label Text and Index"=w931) -> ("Text"=w928:string, "Index"=w929:i32)  [unwired: 12 in, 1 out]
        n370 = Equal?(x=w930, y="Add Item") -> (x = y?=w946:bool)
        n371 = case shown="True" w946 {
          tunnel: w945 -> [_ w970]
          tunnel: w944 -> [_ w968]
          tunnel: w943 -> [_ w969]
          tunnel: [w949 w954] -> w935
          tunnel: [w951 w957] -> w934
          tunnel: w933 -> [w952 _]
          tunnel: T2 {"String"="", "Value"=0} ("Name Value Pair") -> [w953 w956]
          tunnel: w928 -> [_ w955]
          tunnel: w930 -> [w950 _]
          tunnel: w929 -> [w949 w954]
          frame False {
            n372 = Bundle(cluster=w953, "String"=w950, "Value"=w952) -> (w951:T2)
          }
          frame True {
            n373 = control-ref of="Probe Cat Num 01"() -> (w963:refnum<vi>)
            n374 = control-ref of="Probe Cat Num 02"() -> (w966:refnum<vi>)
            n375 = control-ref of="Probe Cat Num 03"() -> (w965:refnum<vi>)
            n376 = control-ref of="Probe Cat Num 04"() -> (w964:refnum<vi>)
            n377 = call "Add New Menu Item.vi"("Base Path"=w968, "Old Value"=w969, "Ring Menu Ref"=w970, "Label or Caption"=w955) -> ("Menu Strings"=w967:string[], "New Item"=w958:string, "Menu Value"=w959:u16)  [unwired: 8 in, 1 out]
            n378 = Bundle(cluster=w956, "String"=w958, "Value"=w959) -> (w957:T2)
            n379 = Build Array(w963, w966, w965, w964) -> (w962:refnum<vi>[])
            n380 = Delete From Array(array=w962, length=1, index=w954) -> (array with subset deleted=w960:refnum<vi>[])  [unwired: 1 out]
            n381 = for {
              tunnel: w960 -> [w972] mode=indexing
              tunnel: w967 -> [w971]
              n382 = property class="Ring (strict)"(reference=w972, "Strings []"=w971) -> ()  [unwired: 1 in, 2 out]
            }
          }
        }
        n383 = Unbundle By Name(w937) -> ("Proble Data"=w940:T3[])
        n384 = Index Array(array=w940, index=w935) -> (element=w941:T3)
        n385 = Bundle By Name(cluster=w941, "Cat Number"=w934) -> (w939:T3)
        n386 = Replace Array Subset(array=w940, new element=w939, index=w935) -> (w938:T3[])
        n387 = Bundle By Name(cluster=w937, "Proble Data"=w938) -> (w936:T1)
      }
      event "Extra Tag 01", "Extra Tag 02", "Extra Tag 03", "Extra Tag 04", "Extra Tag 05", "Extra Tag 06": Value Change {
        n388 = event-data() -> ("OldVal"=w988:u16, "CtlRef"=w987:refnum<vi>)  [unwired: 1 in]
        n389 = property class="Ring (strict)"(reference=w987) -> (reference out=w990:refnum<vi>, "Label.Text"=w977:string, "RingText.Text"=w982:string, "Value"=w981:u16)  [unwired: 1 in, 1 out]
        n390 = call "Get Label Text and Index.vi"("Label Text and Index"=w977) -> ("Text"=w975:string, "Index"=w976:i32)  [unwired: 12 in, 1 out]
        n391 = Equal?(x=w982, y="Add Item") -> (x = y?=w991:bool)
        n392 = case shown="False" w991 {
          tunnel: w990 -> [_ w1017]
          tunnel: w989 -> [_ w1014]
          tunnel: w988 -> [_ w1016]
          tunnel: w975 -> [_ w1015]
          tunnel: [w994 w999] -> w979
          tunnel: [w995 w1003] -> w978
          tunnel: w982 -> [w997 _]
          tunnel: w981 -> [w996 _]
          tunnel: T2 {"String"="", "Value"=0} ("Name Value Pair") -> [w998 w1002]
          tunnel: w976 -> [w994 w999]
          frame False {
            n393 = Bundle(cluster=w998, "String"=w997, "Value"=w996) -> (w995:T2)
          }
          frame True {
            n394 = control-ref of="Extra Tag 01"() -> (w1009:refnum<vi>)
            n395 = control-ref of="Extra Tag 02"() -> (w1012:refnum<vi>)
            n396 = control-ref of="Extra Tag 03"() -> (w1011:refnum<vi>)
            n397 = control-ref of="Extra Tag 04"() -> (w1010:refnum<vi>)
            n398 = control-ref of="Extra Tag 05"() -> (w1001:refnum<vi>)
            n399 = control-ref of="Extra Tag 06"() -> (w1000:refnum<vi>)
            n400 = call "Add New Menu Item.vi"("Base Path"=w1014, "Old Value"=w1016, "Ring Menu Ref"=w1017, "Label or Caption"=w1015) -> ("Menu Strings"=w1013:string[], "New Item"=w1004:string, "Menu Value"=w1005:u16)  [unwired: 8 in, 1 out]
            n401 = Bundle(cluster=w1002, "String"=w1004, "Value"=w1005) -> (w1003:T2)
            n402 = Build Array(w1009, w1012, w1011, w1010, w1001, w1000) -> (w1008:refnum<vi>[])
            n403 = Delete From Array(array=w1008, length=1, index=w999) -> (array with subset deleted=w1006:refnum<vi>[])  [unwired: 1 out]
            n404 = for {
              tunnel: w1006 -> [w1019] mode=indexing
              tunnel: w1013 -> [w1018]
              n405 = property class="Ring (strict)"(reference=w1019, "Strings []"=w1018) -> ()  [unwired: 1 in, 2 out]
            }
          }
        }
        n406 = Unbundle By Name(w984) -> ("Extra Tags"=w986:T2[])
        n407 = Replace Array Subset(array=w986, new element=w978, index=w979) -> (w985:T2[])
        n408 = Bundle By Name(cluster=w984, "Extra Tags"=w985) -> (w983:T1)
      }
      event "Scavenger 01", "Scavenger 02", "Scavenger 03", "Scavenger 04", "Scavenger 05", "Scavenger 06": Value Change {
        n409 = event-data() -> ("OldVal"=w1035:u16, "CtlRef"=w1034:refnum<vi>)  [unwired: 1 in]
        n410 = property class="Ring (strict)"(reference=w1034) -> (reference out=w1037:refnum<vi>, "Label.Text"=w1024:string, "RingText.Text"=w1029:string, "Value"=w1028:u16)  [unwired: 1 in, 1 out]
        n411 = call "Get Label Text and Index.vi"("Label Text and Index"=w1024) -> ("Text"=w1022:string, "Index"=w1023:i32)  [unwired: 12 in, 1 out]
        n412 = Equal?(x=w1029, y="Add Item") -> (x = y?=w1038:bool)
        n413 = case shown="True" w1038 {
          tunnel: w1037 -> [_ w1064]
          tunnel: w1036 -> [_ w1061]
          tunnel: w1035 -> [_ w1063]
          tunnel: w1022 -> [_ w1062]
          tunnel: [w1041 w1046] -> w1026
          tunnel: [w1042 w1050] -> w1025
          tunnel: w1029 -> [w1044 _]
          tunnel: w1028 -> [w1043 _]
          tunnel: T2 {"String"="", "Value"=0} ("Name Value Pair") -> [w1045 w1049]
          tunnel: w1023 -> [w1041 w1046]
          frame False {
            n414 = Bundle(cluster=w1045, "String"=w1044, "Value"=w1043) -> (w1042:T2)
          }
          frame True {
            n415 = control-ref of="Scavenger 01"() -> (w1056:refnum<vi>)
            n416 = control-ref of="Scavenger 02"() -> (w1059:refnum<vi>)
            n417 = control-ref of="Scavenger 03"() -> (w1058:refnum<vi>)
            n418 = control-ref of="Scavenger 04"() -> (w1057:refnum<vi>)
            n419 = control-ref of="Scavenger 05"() -> (w1048:refnum<vi>)
            n420 = control-ref of="Scavenger 06"() -> (w1047:refnum<vi>)
            n421 = call "Add New Menu Item.vi"("Base Path"=w1061, "Old Value"=w1063, "Ring Menu Ref"=w1064, "Label or Caption"=w1062) -> ("Menu Strings"=w1060:string[], "New Item"=w1051:string, "Menu Value"=w1052:u16)  [unwired: 8 in, 1 out]
            n422 = Bundle(cluster=w1049, "String"=w1051, "Value"=w1052) -> (w1050:T2)
            n423 = Build Array(w1056, w1059, w1058, w1057, w1048, w1047) -> (w1055:refnum<vi>[])
            n424 = Delete From Array(array=w1055, length=1, index=w1046) -> (array with subset deleted=w1053:refnum<vi>[])  [unwired: 1 out]
            n425 = for {
              tunnel: w1053 -> [w1066] mode=indexing
              tunnel: w1060 -> [w1065]
              n426 = property class="Ring (strict)"(reference=w1066, "Strings []"=w1065) -> ()  [unwired: 1 in, 2 out]
            }
          }
        }
        n427 = Unbundle By Name(w1031) -> ("Scavenger Tags"=w1033:T2[])
        n428 = Replace Array Subset(array=w1033, new element=w1025, index=w1026) -> (w1032:T2[])
        n429 = Bundle By Name(cluster=w1031, "Scavenger Tags"=w1032) -> (w1030:T1)
      }
      event "Probe Concentration 01", "Probe Concentration 02", "Probe Concentration 03", "Probe Concentration 04": Value Change {
        n430 = event-data() -> ("CtlRef"=w1072:refnum<vi>, "NewVal"=w1069:dbl)  [unwired: 1 in]
        n431 = property class="DigNum (strict)"(reference=w1072) -> ("Label.Text"=w1071:string)  [unwired: 1 in, 2 out]
        n432 = String Length(string=w1071) -> (length=w1078:i32)
        n433 = Subtract(x=w1078, y=2) -> (x-y=w1076:i32)
        n434 = To Unsigned Long Integer(number=w1076) -> (unsigned 32bit integer=w1075:u32)
        n435 = Unbundle By Name(w1080) -> ("Proble Data"=w1083:T3[])
        n436 = Scan From String(input string=w1071, initial scan location=w1075, default 1=0 ("y")) -> (output 1=w1073:i32)  [unwired: 2 in, 3 out]
        n437 = Decrement(x=w1073) -> (x-1=w1070:i32)
        n438 = Index Array(array=w1083, index=w1070) -> (element=w1084:T3)
        n439 = Bundle By Name(cluster=w1084, "Concentration"=w1069) -> (w1082:T3)
        n440 = Replace Array Subset(array=w1083, new element=w1082, index=w1070) -> (w1081:T3[])
        n441 = Bundle By Name(cluster=w1080, "Proble Data"=w1081) -> (w1079:T1)
      }
      event "Buffer Type", "Sample Holder", "Sealant": Value Change {
        n442 = event-data() -> ("OldVal"=w1095:u16, "CtlRef"=w1096:refnum<vi>)  [unwired: 1 in]
        n443 = property class="Ring (strict)"(reference=w1096) -> (reference out=w1098:refnum<vi>, "Label.Text"=w1089:string, "RingText.Text"=w1093:string, "Value"=w1097:u16)  [unwired: 1 in, 1 out]
        n444 = Equal?(x=w1093, y="Add Item") -> (x = y?=w1099:bool)
        n445 = case shown="True" w1099 {
          tunnel: w1098 -> [_ w1124]
          tunnel: w1094 -> [_ w1126]
          tunnel: w1095 -> [_ w1125]
          tunnel: w1089 -> [_ w1123]
          tunnel: w1093 -> [w1118 _]
          tunnel: w1097 -> [w1117 _]
          tunnel: [w1116 w1120] -> w1092
          tunnel: T2 {"String"="", "Value"=0} ("Name Value Pair") -> [w1115 w1119]
          frame False {
            n446 = Bundle(cluster=w1115, "String"=w1118, "Value"=w1117) -> (w1116:T2)
          }
          frame True {
            n447 = call "Add New Menu Item.vi"("Base Path"=w1126, "Old Value"=w1125, "Ring Menu Ref"=w1124, "Label or Caption"=w1123) -> ("New Item"=w1122:string, "Menu Value"=w1121:u16)  [unwired: 8 in, 2 out]
            n448 = Bundle(cluster=w1119, "String"=w1122, "Value"=w1121) -> (w1120:T2)
          }
        }
        n449 = case shown="\"Sample Holder\"" w1089 {
          tunnel: w1092 -> [_ w1104 w1108 w1111 w1114]
          tunnel: w1091 -> [w1102 w1105 w1107 w1110 w1113]
          tunnel: [w1102 w1103 w1106 w1109 w1112] -> w1090
          frame Default {
          }
          frame "Buffer Type" {
            n450 = Bundle By Name(cluster=w1105, "Buffer Type"=w1104) -> (w1103:T1)
          }
          frame "Oxygen Scavenger" {
            n451 = Bundle By Name(cluster=w1107, "Oxygen Scavenger"=w1108) -> (w1106:T1)
          }
          frame "Sample Holder" {
            n452 = Bundle By Name(cluster=w1110, "Sample Holder"=w1111) -> (w1109:T1)
          }
          frame "Sealant" {
            n453 = Bundle By Name(cluster=w1113, "Sealant"=w1114) -> (w1112:T1)
          }
        }
      }
      event "Buffer PH": Value Change {
        n454 = event-data() -> ("NewVal"=w1130:dbl)  [unwired: 1 in]
        n455 = Bundle By Name(cluster=w1131, "Buffer PH"=w1130) -> (w1129:T1)
      }
      event "Notes": Value Change {
        n456 = event-data() -> ("NewVal"=w1136:string)  [unwired: 1 in]
        n457 = Bundle By Name(cluster=w1137, "Notes"=w1136) -> (w1135:T1)
      }
      event "Preset Metadata", "Load Preset": Value Change {
        n458 = event-data() -> ("CtlRef"=w1157:refnum<vi>)  [unwired: 1 in]
        n459 = property class="Ctl"(reference=w1157) -> (reference out=w1155:refnum<vi>, "Label.Text"=w1156:string)  [unwired: 1 in, 1 out]
        n460 = control-ref of="This VI"() -> (w1154:refnum<vi>)
        n461 = property class="VI"(reference=w1154) -> (error out=w1152:errorcluster, "Panel"=w1153:refnum<vi>)  [unwired: 1 in, 1 out]
        n462 = property class="Pnl"(reference=w1153, error in=w1152) -> (error out=w1151:errorcluster, "Controls[]"=w1150:refnum<vi>[])  [unwired: 1 out]
        n463 = case shown="\"Load Preset\", Default" w1156 {
          tunnel: w1158 -> [w1503 w1514]
          tunnel: w1155 -> [_ w1512]
          tunnel: w1151 -> [w1502 w1509]
          tunnel: [w1501 w1507] -> w1143
          tunnel: [w1500 w1506] -> w1142
          frame "Load Preset", Default {
            n464 = call "File Dialog"("start path"=w1503, "prompt"="Select Metadata File", "error in"=w1502, "pattern label"="*.json") -> ("selected path"=w1501:path, "error out"=w1500:errorcluster)  [unwired: 8 in, 2 out]
          }
          frame "Preset Metadata" {
            w1511 = refnum<vi> refnum  # Ring
            n465 = To More Specific Class(target class=w1511, reference=w1512) -> (specific class reference=w1510:refnum<vi>)  [unwired: 1 in, 1 out]
            n466 = property class="Ring"(reference=w1510, error in=w1509) -> (error out=w1506:errorcluster, "RingText.Text"=w1508:string)  [unwired: 1 out]
            n467 = Concatenate Strings(w1508, ".json" ("string")) -> (w1513:string)
            n468 = Build Path(base path=w1514, name or relative path=w1513) -> (appended path=w1507:path)
          }
        }
        n469 = Read from Text File(file (use dialog)=w1143, error in=w1142) -> (text=w1145:string, error out=w1144:errorcluster)  [unwired: 2 in, 2 out]
        n470 = Unflatten From JSON(JSON string=w1145, type and defaults=w1140, error in (no error)=w1144) -> (value=w1141:T1, error out=w1139:errorcluster)  [unwired: 4 in]
        n471 = case shown="No Error" w1139 {
          tunnel: [w1160 w1499] -> w1148
          tunnel: w1150 -> [w1162 _]
          tunnel: w1149 -> [w1161 _]
          tunnel: w1140 -> [_ w1499]
          tunnel: w1141 -> [w1160 _]
          frame No Error {
            n472 = for {
              tunnel: w1162 -> [w1169] mode=indexing
              tunnel: w1160 -> [w1167]
              tunnel: w1161 -> [w1166]
              n473 = property class="Ctl"(reference=w1169) -> (reference out=w1168:refnum<vi>, "Label.Text"=w1165:string)  [unwired: 1 in, 1 out]
              n474 = call "Get Label Text and Index.vi"("Label Text and Index"=w1165) -> ("Label Text and Index (Dup)"=w1164:string, "Index"=w1163:i32)  [unwired: 12 in, 1 out]
              n475 = case shown="\"Scavenger 01\", \"Scavenger 02\", \"Scavenger 03\", \"Scavenger 04\", \"Scavenger 05\", \"Scavenger 06\"" w1164 {
                tunnel: w1168 -> [_ w1178 w1313 w1319 w1325 w1331 w1337 w1343 w1349 w1364 w1384 w1404 w1424 w1436 w1445 w1454 w1463 w1472 w1481 w1490 w1496]
                tunnel: w1167 -> [_ w1176 w1311 w1317 w1323 w1329 w1335 w1341 w1347 w1368 w1388 w1408 w1428 w1439 w1448 w1457 w1466 w1475 w1484 w1493 w1495]
                tunnel: w1166 -> [_ _ w1301 _ _ _ _ _ _ _ _ _ _ _ _ _ _ _ _ _ _]
                tunnel: w1163 -> [_ _ _ _ _ _ _ _ _ w1351 w1371 w1391 w1411 w1431 w1440 w1449 w1458 w1467 w1476 w1485 _]
                frame Default {
                }
                frame "Preset Metadata" {
                  w1179 = refnum<vi> refnum  # Ring
                  n476 = Unbundle By Name(w1176) -> ("Preset Name"=w1171:string)
                  n477 = To More Specific Class(target class=w1179, reference=w1178) -> (specific class reference=w1177:refnum<vi>)  [unwired: 1 in, 1 out]
                  n478 = control-ref of="Preset Metadata"() -> (w1173:refnum<vi>)
                  n479 = property class="Ring (strict)"(reference=w1173) -> ("Strings []"=w1174:string[])  [unwired: 1 in, 2 out]
                  n480 = for {
                    tunnel: w1171 -> [w1186]
                    tunnel: w1174 -> [w1184] mode=indexing
                    tunnel: [w1180] -> w1172
                    i -> [w1180]
                    stop <- w1183 stop-if-true
                    n481 = xnode "Match Regular Expression"("input string"=w1184, "regular expression"=w1186, "ignore case? (F)"=FALSE) -> ("whole match"=w1182:string)  [unwired: 3 in, 4 out]
                    n482 = Not Equal?(x=w1182, y="") -> (x != y?=w1183:bool)
                  }
                  n483 = To Unsigned Word Integer(number=w1172) -> (unsigned 16bit integer=w1170:u16)
                  n484 = To Variant(anything=w1170) -> (Variant=w1175:variant)
                  n485 = property class="Ring"(reference=w1177, "Value"=w1175) -> ()  [unwired: 1 in, 2 out]
                }
                frame "Sample Type" {
                  w1314 = refnum<vi> refnum  # Ring
                  n486 = Unbundle By Name(w1311) -> ("Sample Type.Value"=w1310:u16)
                  n487 = To More Specific Class(target class=w1314, reference=w1313) -> (specific class reference=w1312:refnum<vi>)  [unwired: 1 in, 1 out]
                  n488 = To Variant(anything=w1310) -> (Variant=w1309:variant)
                  n489 = property class="Ring"(reference=w1312, "Value"=w1309) -> (reference out=w1308:refnum<vi>)  [unwired: 1 in, 1 out]
                  n490 = property class="Ring"(reference=w1308) -> ("RingText.Text"=w1302:string)  [unwired: 1 in, 2 out]
                  n491 = control-ref of="Sample Type Sub Types"() -> (w1306:refnum<vi>)
                  n492 = call "Populate Sub Menu.vi"("Sample Type Sub Types"=w1306, "Base Path"=w1301, "Ring Text"=w1302) -> ("Sample Type Sub Types (Dup)"=w1305:refnum<vi>, "Caption Text"=w1304:string, "Menu Items"=w1303:string[])  [unwired: 10 in]
                  n493 = property class="Ring (strict)"(reference=w1305, "Caption.Text"=w1304, "Value"=u16 0, "Strings []"=w1303) -> ()  [unwired: 1 in, 2 out]
                }
                frame "Sample Type Sub Types" {
                  w1320 = refnum<vi> refnum  # Ring
                  n494 = Unbundle By Name(w1317) -> ("Sample Sub Type.Value"=w1316:u16)
                  n495 = To More Specific Class(target class=w1320, reference=w1319) -> (specific class reference=w1318:refnum<vi>)  [unwired: 1 in, 1 out]
                  n496 = To Variant(anything=w1316) -> (Variant=w1315:variant)
                  n497 = property class="Ring"(reference=w1318, "Value"=w1315) -> ()  [unwired: 1 in, 2 out]
                }
                frame "Sample Holder" {
                  w1326 = refnum<vi> refnum  # Ring
                  n498 = Unbundle By Name(w1323) -> ("Sample Holder.Value"=w1322:u16)
                  n499 = To More Specific Class(target class=w1326, reference=w1325) -> (specific class reference=w1324:refnum<vi>)  [unwired: 1 in, 1 out]
                  n500 = To Variant(anything=w1322) -> (Variant=w1321:variant)
                  n501 = property class="Ring"(reference=w1324, "Value"=w1321) -> ()  [unwired: 1 in, 2 out]
                }
                frame "Sealant" {
                  w1332 = refnum<vi> refnum  # Ring
                  n502 = Unbundle By Name(w1329) -> ("Sealant.Value"=w1328:u16)
                  n503 = To More Specific Class(target class=w1332, reference=w1331) -> (specific class reference=w1330:refnum<vi>)  [unwired: 1 in, 1 out]
                  n504 = To Variant(anything=w1328) -> (Variant=w1327:variant)
                  n505 = property class="Ring"(reference=w1330, "Value"=w1327) -> ()  [unwired: 1 in, 2 out]
                }
                frame "Buffer Type" {
                  w1338 = refnum<vi> refnum  # Ring
                  n506 = Unbundle By Name(w1335) -> ("Buffer Type.Value"=w1334:u16)
                  n507 = To More Specific Class(target class=w1338, reference=w1337) -> (specific class reference=w1336:refnum<vi>)  [unwired: 1 in, 1 out]
                  n508 = To Variant(anything=w1334) -> (Variant=w1333:variant)
                  n509 = property class="Ring"(reference=w1336, "Value"=w1333) -> ()  [unwired: 1 in, 2 out]
                }
                frame "Oxygen Scavenger" {
                  w1344 = refnum<vi> refnum  # Ring
                  n510 = Unbundle By Name(w1341) -> ("Oxygen Scavenger.Value"=w1340:u16)
                  n511 = To More Specific Class(target class=w1344, reference=w1343) -> (specific class reference=w1342:refnum<vi>)  [unwired: 1 in, 1 out]
                  n512 = To Variant(anything=w1340) -> (Variant=w1339:variant)
                  n513 = property class="Ring"(reference=w1342, "Value"=w1339) -> ()  [unwired: 1 in, 2 out]
                }
                frame "Buffer PH" {
                  w1350 = refnum<vi> refnum  # Numeric
                  n514 = Unbundle By Name(w1347) -> ("Buffer PH"=w1346:dbl)
                  n515 = To More Specific Class(target class=w1350, reference=w1349) -> (specific class reference=w1348:refnum<vi>)  [unwired: 1 in, 1 out]
                  n516 = To Variant(anything=w1346) -> (Variant=w1345:variant)
                  n517 = property class="Num"(reference=w1348, "Value"=w1345) -> ()  [unwired: 1 in, 2 out]
                }
                frame "Probe 1" {
                  w1365 = refnum<vi> refnum  # Boolean
                  n518 = Unbundle By Name(w1368) -> ("Proble Data"=w1367:T3[])
                  n519 = To More Specific Class(target class=w1365, reference=w1364) -> (specific class reference=w1363:refnum<vi>)  [unwired: 1 in, 1 out]
                  n520 = Index Array(array=w1367, index=w1351) -> (element=w1366:T3)
                  n521 = Unbundle By Name(w1366) -> ("Active?"=w1353:bool)
                  n522 = To Variant(anything=w1353) -> (Variant=w1362:variant)
                  n523 = Select(t=T6."Enabled" ("Disabled"), s=w1353, f=T6."Disabled and Grayed Out" ("Disabled")) -> (s? t:f=w1352:T6)
                  n524 = property class="Bool"(reference=w1363, "Value"=w1362) -> ()  [unwired: 1 in, 2 out]
                  n525 = control-ref of="Probe Name 01"() -> (w1358:refnum<vi>)
                  n526 = control-ref of="Image Target 01"() -> (w1359:refnum<vi>)
                  n527 = control-ref of="Probe Sub Type 01"() -> (w1360:refnum<vi>)
                  n528 = control-ref of="Probe Cat Num 01"() -> (w1361:refnum<vi>)
                  n529 = control-ref of="Probe Concentration 01"() -> (w1356:refnum<vi>)
                  n530 = Build Array(w1358, w1359, w1360, w1361) -> (w1357:refnum<vi>[])
                  n531 = for {
                    tunnel: w1357 -> [w1370] mode=indexing
                    tunnel: w1352 -> [w1369]
                    n532 = property class="Ring (strict)"(reference=w1370, "DisabledEnum"=w1369) -> ()  [unwired: 1 in, 2 out]
                  }
                  n533 = property class="DigNum (strict)"(reference=w1356, "DisabledEnum"=w1352) -> ()  [unwired: 1 in, 2 out]
                }
                frame "Probe 2" {
                  w1385 = refnum<vi> refnum  # Boolean
                  n534 = Unbundle By Name(w1388) -> ("Proble Data"=w1387:T3[])
                  n535 = To More Specific Class(target class=w1385, reference=w1384) -> (specific class reference=w1383:refnum<vi>)  [unwired: 1 in, 1 out]
                  n536 = Index Array(array=w1387, index=w1371) -> (element=w1386:T3)
                  n537 = Unbundle By Name(w1386) -> ("Active?"=w1373:bool)
                  n538 = To Variant(anything=w1373) -> (Variant=w1382:variant)
                  n539 = Select(t=T6."Enabled" ("Disabled"), s=w1373, f=T6."Disabled and Grayed Out" ("Disabled")) -> (s? t:f=w1372:T6)
                  n540 = property class="Bool"(reference=w1383, "Value"=w1382) -> ()  [unwired: 1 in, 2 out]
                  n541 = control-ref of="Probe Name 02"() -> (w1378:refnum<vi>)
                  n542 = control-ref of="Image Target 02"() -> (w1379:refnum<vi>)
                  n543 = control-ref of="Probe Sub Type 02"() -> (w1380:refnum<vi>)
                  n544 = control-ref of="Probe Cat Num 02"() -> (w1381:refnum<vi>)
                  n545 = control-ref of="Probe Concentration 02"() -> (w1376:refnum<vi>)
                  n546 = Build Array(w1378, w1379, w1380, w1381) -> (w1377:refnum<vi>[])
                  n547 = for {
                    tunnel: w1377 -> [w1390] mode=indexing
                    tunnel: w1372 -> [w1389]
                    n548 = property class="Ring (strict)"(reference=w1390, "DisabledEnum"=w1389) -> ()  [unwired: 1 in, 2 out]
                  }
                  n549 = property class="DigNum (strict)"(reference=w1376, "DisabledEnum"=w1372) -> ()  [unwired: 1 in, 2 out]
                }
                frame "Probe 3" {
                  w1405 = refnum<vi> refnum  # Boolean
                  n550 = Unbundle By Name(w1408) -> ("Proble Data"=w1407:T3[])
                  n551 = To More Specific Class(target class=w1405, reference=w1404) -> (specific class reference=w1403:refnum<vi>)  [unwired: 1 in, 1 out]
                  n552 = Index Array(array=w1407, index=w1391) -> (element=w1406:T3)
                  n553 = Unbundle By Name(w1406) -> ("Active?"=w1393:bool)
                  n554 = To Variant(anything=w1393) -> (Variant=w1402:variant)
                  n555 = Select(t=T6."Enabled" ("Disabled"), s=w1393, f=T6."Disabled and Grayed Out" ("Disabled")) -> (s? t:f=w1392:T6)
                  n556 = property class="Bool"(reference=w1403, "Value"=w1402) -> ()  [unwired: 1 in, 2 out]
                  n557 = control-ref of="Probe Name 03"() -> (w1398:refnum<vi>)
                  n558 = control-ref of="Image Target 03"() -> (w1399:refnum<vi>)
                  n559 = control-ref of="Probe Sub Type 03"() -> (w1400:refnum<vi>)
                  n560 = control-ref of="Probe Cat Num 03"() -> (w1401:refnum<vi>)
                  n561 = control-ref of="Probe Concentration 03"() -> (w1396:refnum<vi>)
                  n562 = Build Array(w1398, w1399, w1400, w1401) -> (w1397:refnum<vi>[])
                  n563 = for {
                    tunnel: w1397 -> [w1410] mode=indexing
                    tunnel: w1392 -> [w1409]
                    n564 = property class="Ring (strict)"(reference=w1410, "DisabledEnum"=w1409) -> ()  [unwired: 1 in, 2 out]
                  }
                  n565 = property class="DigNum (strict)"(reference=w1396, "DisabledEnum"=w1392) -> ()  [unwired: 1 in, 2 out]
                }
                frame "Probe 4" {
                  w1425 = refnum<vi> refnum  # Boolean
                  n566 = Unbundle By Name(w1428) -> ("Proble Data"=w1427:T3[])
                  n567 = To More Specific Class(target class=w1425, reference=w1424) -> (specific class reference=w1423:refnum<vi>)  [unwired: 1 in, 1 out]
                  n568 = Index Array(array=w1427, index=w1411) -> (element=w1426:T3)
                  n569 = Unbundle By Name(w1426) -> ("Active?"=w1413:bool)
                  n570 = To Variant(anything=w1413) -> (Variant=w1422:variant)
                  n571 = Select(t=T6."Enabled" ("Disabled"), s=w1413, f=T6."Disabled and Grayed Out" ("Disabled")) -> (s? t:f=w1412:T6)
                  n572 = property class="Bool"(reference=w1423, "Value"=w1422) -> ()  [unwired: 1 in, 2 out]
                  n573 = control-ref of="Probe Name 04"() -> (w1418:refnum<vi>)
                  n574 = control-ref of="Image Target 04"() -> (w1419:refnum<vi>)
                  n575 = control-ref of="Probe Sub Type 04"() -> (w1420:refnum<vi>)
                  n576 = control-ref of="Probe Cat Num 04"() -> (w1421:refnum<vi>)
                  n577 = control-ref of="Probe Concentration 04"() -> (w1416:refnum<vi>)
                  n578 = Build Array(w1418, w1419, w1420, w1421) -> (w1417:refnum<vi>[])
                  n579 = for {
                    tunnel: w1417 -> [w1430] mode=indexing
                    tunnel: w1412 -> [w1429]
                    n580 = property class="Ring (strict)"(reference=w1430, "DisabledEnum"=w1429) -> ()  [unwired: 1 in, 2 out]
                  }
                  n581 = property class="DigNum (strict)"(reference=w1416, "DisabledEnum"=w1412) -> ()  [unwired: 1 in, 2 out]
                }
                frame "Probe Name 01", "Probe Name 02", "Probe Name 03", "Probe Name 04" {
                  w1432 = refnum<vi> refnum  # Ring
                  n582 = Unbundle By Name(w1439) -> ("Proble Data"=w1438:T3[])
                  n583 = To More Specific Class(target class=w1432, reference=w1436) -> (specific class reference=w1435:refnum<vi>)  [unwired: 1 in, 1 out]
                  n584 = Index Array(array=w1438, index=w1431) -> (element=w1437:T3)
                  n585 = Unbundle By Name(w1437) -> ("Name.Value"=w1433:u16)
                  n586 = To Variant(anything=w1433) -> (Variant=w1434:variant)
                  n587 = property class="Ring"(reference=w1435, "Value"=w1434) -> ()  [unwired: 1 in, 2 out]
                }
                frame "Image Target 01", "Image Target 02", "Image Target 03", "Image Target 04" {
                  w1441 = refnum<vi> refnum  # Ring
                  n588 = Unbundle By Name(w1448) -> ("Proble Data"=w1447:T3[])
                  n589 = To More Specific Class(target class=w1441, reference=w1445) -> (specific class reference=w1444:refnum<vi>)  [unwired: 1 in, 1 out]
                  n590 = Index Array(array=w1447, index=w1440) -> (element=w1446:T3)
                  n591 = Unbundle By Name(w1446) -> ("Target.Value"=w1442:u16)
                  n592 = To Variant(anything=w1442) -> (Variant=w1443:variant)
                  n593 = property class="Ring"(reference=w1444, "Value"=w1443) -> ()  [unwired: 1 in, 2 out]
                }
                frame "Probe Sub Type 01", "Probe Sub Type 02", "Probe Sub Type 03", "Probe Sub Type 04" {
                  w1450 = refnum<vi> refnum  # Ring
                  n594 = Unbundle By Name(w1457) -> ("Proble Data"=w1456:T3[])
                  n595 = To More Specific Class(target class=w1450, reference=w1454) -> (specific class reference=w1453:refnum<vi>)  [unwired: 1 in, 1 out]
                  n596 = Index Array(array=w1456, index=w1449) -> (element=w1455:T3)
                  n597 = Unbundle By Name(w1455) -> ("Sub Type.Value"=w1451:u16)
                  n598 = To Variant(anything=w1451) -> (Variant=w1452:variant)
                  n599 = property class="Ring"(reference=w1453, "Value"=w1452) -> ()  [unwired: 1 in, 2 out]
                }
                frame "Probe Cat Num 01", "Probe Cat Num 02", "Probe Cat Num 03", "Probe Cat Num 04" {
                  w1459 = refnum<vi> refnum  # Ring
                  n600 = Unbundle By Name(w1466) -> ("Proble Data"=w1465:T3[])
                  n601 = To More Specific Class(target class=w1459, reference=w1463) -> (specific class reference=w1462:refnum<vi>)  [unwired: 1 in, 1 out]
                  n602 = Index Array(array=w1465, index=w1458) -> (element=w1464:T3)
                  n603 = Unbundle By Name(w1464) -> ("Cat Number.Value"=w1460:u16)
                  n604 = To Variant(anything=w1460) -> (Variant=w1461:variant)
                  n605 = property class="Ring"(reference=w1462, "Value"=w1461) -> ()  [unwired: 1 in, 2 out]
                }
                frame "Probe Concentration 01", "Probe Concentration 02", "Probe Concentration 03", "Probe Concentration 04" {
                  w1468 = refnum<vi> refnum  # Numeric
                  n606 = Unbundle By Name(w1475) -> ("Proble Data"=w1474:T3[])
                  n607 = To More Specific Class(target class=w1468, reference=w1472) -> (specific class reference=w1471:refnum<vi>)  [unwired: 1 in, 1 out]
                  n608 = Index Array(array=w1474, index=w1467) -> (element=w1473:T3)
                  n609 = Unbundle By Name(w1473) -> ("Concentration"=w1469:dbl)
                  n610 = To Variant(anything=w1469) -> (Variant=w1470:variant)
                  n611 = property class="Num"(reference=w1471, "Value"=w1470) -> ()  [unwired: 1 in, 2 out]
                }
                frame "Extra Tag 01", "Extra Tag 02", "Extra Tag 03", "Extra Tag 04", "Extra Tag 05", "Extra Tag 06" {
                  w1477 = refnum<vi> refnum  # Ring
                  n612 = Unbundle By Name(w1484) -> ("Extra Tags"=w1483:T2[])
                  n613 = To More Specific Class(target class=w1477, reference=w1481) -> (specific class reference=w1480:refnum<vi>)  [unwired: 1 in, 1 out]
                  n614 = Index Array(array=w1483, index=w1476) -> (element=w1482:T2)
                  n615 = Unbundle By Name(w1482) -> ("Value"=w1478:u16)
                  n616 = To Variant(anything=w1478) -> (Variant=w1479:variant)
                  n617 = property class="Ring"(reference=w1480, "Value"=w1479) -> ()  [unwired: 1 in, 2 out]
                }
                frame "Scavenger 01", "Scavenger 02", "Scavenger 03", "Scavenger 04", "Scavenger 05", "Scavenger 06" {
                  w1486 = refnum<vi> refnum  # Ring
                  n618 = Unbundle By Name(w1493) -> ("Scavenger Tags"=w1492:T2[])
                  n619 = To More Specific Class(target class=w1486, reference=w1490) -> (specific class reference=w1489:refnum<vi>)  [unwired: 1 in, 1 out]
                  n620 = Index Array(array=w1492, index=w1485) -> (element=w1491:T2)
                  n621 = Unbundle By Name(w1491) -> ("Value"=w1487:u16)
                  n622 = To Variant(anything=w1487) -> (Variant=w1488:variant)
                  n623 = property class="Ring"(reference=w1489, "Value"=w1488) -> ()  [unwired: 1 in, 2 out]
                }
                frame "Notes" {
                  w1497 = refnum<vi> refnum  # String
                  n624 = Unbundle By Name(w1495) -> ("Notes"=w1494:string)
                  n625 = To More Specific Class(target class=w1497, reference=w1496) -> (specific class reference=w1498:refnum<vi>)  [unwired: 1 in, 1 out]
                  n626 = property class="Str"(reference=w1498, "Value"=w1494) -> ()  [unwired: 1 in, 2 out]
                }
              }
            }
          }
          frame Error {
          }
        }
      }
      event "Save New Preset": Value Change {
        n627 = event-data() -> ()  [unwired: 1 in, 1 out]
        n628 = call "Get User Input.vi"("Dialog Message"="Metadata Preset Name") -> ("User Input"=w1520:string, "Canceled?"=w1521:bool)  [unwired: 13 in]
        n629 = case shown="False" w1521 {
          tunnel: w1523 -> [w1540 _]
          tunnel: w1520 -> [w1531 _]
          tunnel: w1519 -> [w1539 w1666]
          tunnel: [w1537 w1666] -> w1518
          frame False {
            n630 = control-ref of="Preset Metadata"() -> (w1541:refnum<vi>)
            n631 = Concatenate Strings(w1531, ".json" ("string")) -> (w1543:string)
            n632 = property class="Ring (strict)"(reference=w1541) -> (reference out=w1535:refnum<vi>, "Strings []"=w1530:string[])  [unwired: 1 in, 1 out]
            n633 = Build Path(base path=w1540, name or relative path=w1543) -> (appended path=w1538:path)
            n634 = Bundle By Name(cluster=w1539, "Preset Name"=w1531) -> (w1537:T1)
            n635 = Split 1D Array(array=w1530, index=1) -> (first subarray=w1527:string[], second subarray=w1528:string[])
            n636 = Flatten To JSON(anything=w1537) -> (JSON string=w1544:string)  [unwired: 2 in, 1 out]
            n637 = Write to Text File(file (use dialog)=w1538, text=w1544) -> ()  [unwired: 2 in, 3 out]
            n638 = Build Array (concatenate)(w1528, w1531) -> (w1536:string[])
            n639 = call "Sorry String Array.vi"("Array of String"=w1536) -> ("Sorted Array"=w1526:string[])  [unwired: 14 in]
            n640 = Build Array (concatenate)(w1527, w1526) -> (w1525:string[])
            n641 = for {
              tunnel: w1531 -> [w1551]
              tunnel: w1525 -> [w1549] mode=indexing
              tunnel: [w1545] -> w1533
              i -> [w1545]
              stop <- w1548 stop-if-true
              n642 = xnode "Match Regular Expression"("input string"=w1549, "regular expression"=w1551, "ignore case? (F)"=FALSE) -> ("whole match"=w1547:string)  [unwired: 3 in, 4 out]
              n643 = Not Equal?(x=w1547, y="") -> (x != y?=w1548:bool)
            }
            n644 = property class="Ring (strict)"(reference=w1535, "Strings []"=w1525) -> (reference out=w1534:refnum<vi>)  [unwired: 1 in, 1 out]
            n645 = To Unsigned Word Integer(number=w1533) -> (unsigned 16bit integer=w1532:u16)
            n646 = property class="Ring (strict)"(reference=w1534, "Value"=w1532) -> ()  [unwired: 1 in, 2 out]
          }
          frame True {
          }
        }
      }
      event "Save": Value Change {
        n647 = event-data() -> ("NewVal"=w1696:bool)  [unwired: 1 in]
        n648 = Strip Path(path=w1679) -> (stripped path=w1673:path)  [unwired: 1 out]
        n649 = Build Path(base path=w1673, name or relative path="Last File.json") -> (appended path=w1670:path)
        n650 = property on="Dirty Quit" class="Bool (strict)"("Val(Sgnl)"=TRUE ("Value (Signaling)")) -> ()  [unwired: 2 in, 2 out]
        n651 = Path To String(path=w1667) -> (string=w1671:string)
        n652 = Build Path(base path=w1673, name or relative path="Last Used.json") -> (appended path=w1693:path)
        n653 = Write to Text File(file (use dialog)=w1670, text=w1671) -> (error out=→"Last File Write Error":errorcluster)  [unwired: 2 in, 2 out]
        n654 = Flatten To JSON(anything=w1694) -> (JSON string=w1675:string, 11:w1678:errorcluster)  [unwired: 2 in]
        n655 = Write to Text File(file (use dialog)=w1693, text=w1675, error in=w1678) -> (error out=w1677:errorcluster)  [unwired: 1 in, 2 out]
        n656 = Strip Path(path=w1667) -> (stripped path=w1682:path)  [unwired: 1 out]
        n657 = Concatenate Strings(w1668, "_" ("string"), "Sample Metadata.json" ("name or relative path")) -> (w1692:string)
        n658 = call <vilib>:"Check if File or Folder Exists.vi"("error in (no error)"=w1677, "path"=w1682) -> ("error out"=w1683:errorcluster, "file or folder exists?"=w1685:bool, "dup path"=w1684:path)  [unwired: 7 in]
        n659 = case shown="False" w1685 {
          tunnel: w1684 -> [w1709 w1711]
          tunnel: [w1708 w1711] -> w1681
          tunnel: w1683 -> [w1707 w1710]
          tunnel: [w1706 w1710] -> w1676
          frame False {
            n660 = Create Folder(path (use dialog)=w1709, error in=w1707) -> (created path=w1708:path, error out=w1706:errorcluster)  [unwired: 1 in, 1 out]
          }
          frame True {
          }
        }
        n661 = Build Path(base path=w1681, name or relative path=w1692) -> (appended path=w1690:path)
        n662 = Write to Text File(file (use dialog)=w1690, text=w1675, error in=w1676) -> (error out=w1680:errorcluster)  [unwired: 1 in, 2 out]
        n663 = case shown="No Error" w1680 {
          tunnel: w1675 -> [_ w1705]
          frame No Error {
          }
          frame Error {
            w1701 = 0 items=["Desktop"=0, "Personal Documents"=5, "AppData"=26, "Local AppData"=28, "Common AppData"=35, "Program Files"=38, "Program Files Common"=43, "Common Documents"=46] ("Requested Path")
            w1702 = 0 ("HWND")
            n664 = call "Sample Metadata Get Date Time String.vi"() -> ("Date Time String"=w1698:string)  [unwired: 15 in]
            n665 = dll-call lib="shell32.dll" fn="SHGetFolderPathA"("HWND"=w1702, "nFolder"=w1701, "hToken"=w1702, "dwFlags"=w1702) -> ("pszPath"=w1703:string)  [unwired: 9 in, 2 out]
            n666 = Concatenate Strings(w1698, " Sample Metadata.json" ("string")) -> (w1697:string)
            n667 = String To Path(string=w1703) -> (path=w1704:path)
            n668 = Build Path(base path=w1704, name or relative path=w1697) -> (appended path=w1700:path)
            n669 = Write to Text File(file (use dialog)=w1700, text=w1705) -> ()  [unwired: 2 in, 3 out]
          }
        }
        n670 = Merge Errors(w1680, w1689) -> (w1688:errorcluster)
        "File Path (Dup)" <- w1667
      }
    }
  }
  "Write Error" <- w24
  "Canceled?" <- w23
  n671 = property class="Pnl"(reference=w15, error in=w16) -> (error out=w12:errorcluster, "Controls[]"=w14:refnum<vi>[])  [unwired: 1 out]
  n672 = To Word Integer(number=w78) -> (16bit integer=w80:i16)
  n673 = To Word Integer(number=w81) -> ()  [unwired: 1 out]
  n674 = property class="Bool"(reference=w65) -> ("Height"=w83:u32, "Top"=w84:i32)  [unwired: 1 in, 2 out]
  n675 = Unbundle By Name(w75) -> ("Left"=w77:i16, "Top"=w88:i16)
  n676 = register-events(error in=w12, w14) -> (reference out=w13:refnum<event-registration>, error out=w11:errorcluster)  [unwired: 1 in]
  n677 = To Word Integer(number=w83) -> (16bit integer=w86:i16)
  n678 = To Word Integer(number=w84) -> (16bit integer=w87:i16)
  n679 = Add(x=w77, y=w80) -> (x+y=w79:i16)
  n680 = while {
    tunnel: w13 -> [w1715]
    tunnel: w11 -> [w1714]
    tunnel: [w1712] -> w10
    stop <- w1713 stop-if-true
    n681 = event shown="[1] \"Dirty Quit\": Value Change" {
      selector: w1715 -> [_ _]
      dyn-events: [_ _] -> w1712
      timeout: _ -> [_ _]
      tunnel: w1714 -> [_ _]
      tunnel: [FALSE ("NewVal") w1728] -> w1713
      event Value Change {
        n682 = event-data() -> ("CtlRef"=w1725:refnum<vi>)  [unwired: 1 out]
        n683 = property class="Ctl"(reference=w1725) -> ("Label.Text"=w1720:string)  [unwired: 1 in, 2 out]
        n684 = Not Equal?(x=w1720, y="Preset Metadata") -> (x != y?=w1719:bool)
        n685 = Not Equal?(x=w1720, y="Load Preset") -> (x != y?=w1717:bool)
        n686 = Not Equal?(x=w1720, y="Save New Preset") -> (x != y?=w1718:bool)
        n687 = Compound Arithmetic op=AND(w1719, w1717, w1718) -> (w1716:bool)
        n688 = case shown="True" w1716 {
          frame False {
          }
          frame True {
            n689 = control-ref of="Preset Metadata"() -> (w1726:refnum<vi>)
            n690 = property class="Ring (strict)"(reference=w1726, "Value"=u16 0) -> ()  [unwired: 1 in, 2 out]
          }
        }
      }
      event "Dirty Quit": Value Change {
        n691 = event-data() -> ("NewVal"=w1728:bool)  [unwired: 1 out]
      }
    }
  }
  n692 = Compound Arithmetic op=ADD(w88, w86, w87, i16 12 ("y")) -> (w82:i16)
  n693 = Bundle By Name(cluster=w75, "Right"=w79, "Bottom"=w82) -> (w76:T7)
  n694 = property class="VI"(reference=w74, "Front Panel.PanelBounds"=w76, "Front Panel.IsFrontmost"=TRUE ("Front Panel Window:Is Frontmost")) -> (reference out=w58:refnum<vi>)  [unwired: 1 in, 1 out]
  n695 = invoke class="VI" method="FP.Center"(reference=w58) -> ()  [unwired: 2 in, 3 out]
  n696 = Unregister For Events(event registration refnum=w10) -> ()  [unwired: 1 in, 1 out]
